vi "OCU_Lyras.vi"(9 "Overview Image Ref In":T7, 10 "at":T6="LPB Pool", 11 "Location of THINK":T11="127.0.0.1") -> ()   [LabVIEW 2013]
doc: "This is the current implementation of the operator control unit (OCU) for sailbot interfacing with this OCU over a network connection. The following features are currently implemented:\n- override control of the rudden angle and sail value by control interface or using keys\n- ability to add missions before and during a run, by clicking and by using GPS location of the boat or an auxiliary GPS attached to the OCU computer\n- modification of tuning values used on the boat\n- indicators for all relevant system status information\n\nAuthors: Jared Kirschner, Jason Curtis"
uses:
  trunk/Software/2-Think/2 Typedefs/sail setpt.ctl
  trunk/Software/2-Think/2 Typedefs/rudder angle.ctl
  trunk/Software/2-Think/2 Typedefs/setpoints to boat.ctl
  trunk/Software/0x2-OCU-Think Comm/0x2 Typedefs/manual override.ctl
  trunk/Software/2-Think/2 Typedefs/eStopCommand.ctl
  trunk/Software/0x2-OCU-Think Comm/0x2 Typedefs/Current Waypoint.ctl
  cRIO_Code/Data/TypeDefs/UTM Location.ctl
  RIO-OCU_Comm/NetworkStreams/Reader/NetworkStreamReader.lvclass
  RIO-OCU_Comm/NetworkStreams/Reader/readType.ctl
  trunk/Software/0x2-OCU-Think Comm/0x2 Typedefs/ocuMessage.ctl
  trunk/Software/0x2-OCU-Think Comm/0x2 Typedefs/ocuCommands.ctl
  RIO-OCU_Comm/NetworkStreams/Writer/NetworkStreamWriter.lvclass
  trunk/Software/2-Think/2 Typedefs/indicator LED.ctl
  trunk/Software/2-Think/2 Typedefs/generalized sensor status.ctl
  trunk/Software/2-Think/2 Typedefs/generalized actuator status.ctl
  trunk/Software/2-Think/2 Typedefs/Which Boat.ctl
  trunk/Software/2-Think/2 Typedefs/robot velocity.ctl
  trunk/Software/2-Think/2 Typedefs/heading.ctl
  trunk/Software/2-Think/2 Typedefs/rate of turn.ctl
  trunk/Software/2-Think/2 Typedefs/pitch and roll.ctl
  trunk/Software/2-Think/2 Typedefs/apparent wind.ctl
  trunk/Software/2-Think/2 Typedefs/apparent wind speed.ctl
  trunk/Software/2-Think/2 Typedefs/apparent wind direction.ctl
  trunk/Software/2-Think/2 Typedefs/Velocity.ctl
  trunk/Software/2-Think/2 Typedefs/absolute wind direction.ctl
  trunk/Software/2-Think/2 Typedefs/absolute wind speed.ctl
  trunk/Software/2-Think/2 Typedefs/absolute water current vector.ctl
  trunk/Software/0x2-OCU-Think Comm/0x2 Typedefs/RIO-OCU update controls.ctl
  trunk/Software/0-OCU/0 Typedefs/Mission Type Radio Buttons.ctl
  trunk/Software/2-Think/2 Typedefs/Goodness Fns Indicator.ctl
  trunk/Software/2-Think/2 Typedefs/UTM Circle.ctl
  trunk/Software/2-Think/2 Globals/2 Global.vi
  trunk/Software/2-Think/2 Typedefs/tacking attempt.ctl
  OCU/Location of Think.ctl
  trunk/Software/0x2-OCU-Think Comm/OCUtoSim.vi
  cRIO_Code/Logic/Classes/Missions/GenericMission/GenericMission.lvclass
  trunk/Software/0-OCU/0 Typedefs/Sail Position.ctl
  trunk/Software/0-OCU/0 Typedefs/Rudder Position.ctl
  trunk/Software/0-OCU/0 Typedefs/Apparent Wind Point of Sail.ctl
  cRIO_Code/Data/TypeDefs/ocuWaypoint.ctl
  cRIO_Code/Logic/Classes/Waypoint/Waypoint.lvclass
  cRIO_Code/Data/TypeDefs/Waypoints List.ctl
  trunk/Software/2-Think/2 Typedefs/PI Constants.ctl
  trunk/Software/2-Think/2 Typedefs/Goodness Weightings.ctl
  trunk/Software/0-OCU/0 Typedefs/Maps.ctl
  <vilib>/vision/Image Controls.llb/IMAQ Image.ctl
  trunk/Software/0x2-OCU-Think Comm/0x2 Typedefs/Sail Setting Tuning.ctl
  trunk/Software/0x2-OCU-Think Comm/0x2 Typedefs/Control values.ctl
panel:
  in  "Tab Control":T1(tab)
  out "Sail Position 2":T2 scale=1.0..-1.0
  out "Rudder Position":T3 scale=50.0..-50.0 scale format="%#_2f"
  in  "Mission Entry Type":T4
  in  "Tolerance":dbl=3.0
  in  "Time(s)":dbl=300.0
  out "You are sailing":T5
  out "Battery Voltage":dbl
  out "Connected?":bool caption="Connection Status"
  out "Mission Map":T7(plugin-control)
  out "# of Waypts":i32
  in  "Overlay Font Size":i16=40
  in  "Stop":bool
  in  "Map Mode":enum32{"M[i]ssion Edit", "M[o]nitoring"}(tab)
  in  "Load MDF":bool
  in  "Mission Def Filepath":path caption="MDF (Mission Definition File) path"
  in  "Reset Missions/Waypts":bool
  in  "Save Waypoints\nand PoI":bool
  out "Absolute\nWind\nDirection":dbl
  out "Heading":T8 format="%05.1f"
  in  "Plot Colors":T9={"Target"=3381759, "No Sail"=16711680, "Change"=16756736, "Pure Waypt"=35080, "Pure Wind"=16860, "Combined"=16777228}
  out "Goodness Functions":picture
  out "Apparent Wind Direction\nPoint of Sail":T10 scale=0.0..360.0 scale format="%4d"
  out "Mission Status":string caption="Current Mission\nStatus"
  in  "GPS COM port":refnum<visa-resource-name>="COM1"
  out "Sensor Status":T12
  in  "Enable \nLocal GPS":bool
  out "Local Wind":dbl
  in  "Log message":string caption="Log message (type and press enter)"
  out "Mission Map 2":T7(plugin-control)
  out "# of Waypts 2":i32
  in  "Overlay Font Size 2":i16=40
  in  "Save Image":bool
  in  "OVERRIDE SAIL?":bool
  in  "OVERRIDE RUDDER?":bool
  in  "Globals":T14(tab)
  out "Don't Tip?":bool
  out "Wind Sensor Status":T12
  out "Estimated Error":dbl
  out "Robot Heading":T8 format="%05.1f"
  out "Robot UTM Location":T15 {"North" format="%#_10f"; "East" format="%#_8f"}
  out "Robot Velocity":T16
  out "Robot\nRate of Turn":T17 format="%05.1f"
  out "Robot Pitch/Roll":T18 {"Roll" format="%05.1f"; "Pitch" format="%05.1f"}
  out "Robot Speed (m/s)":dbl
  out "Absolute Wind":T19 {"East" format="%#_5g"}
  out "Apparent Wind Direction":T20
  out "Apparent Wind Speed":T21
  out "Apparent Wind":T22
  out "Crossing Wind":bool
  out "Setpoints to boat":T23
  out "Sail Position":T24
  out "Rudder Angle":T25
  out "Current Waypoint":T26
  in  "Reset to start":bool
  out "Manual Override":T27
  out "Waypoints Array":T28[](array[typedef]) {"UTM Location"."North" format="%#_10f"; "UTM Location"."East" format="%#_8f"}
  out "Waypoints Object Array":T29
  out "Mission Object Array":refnum<class "GenericMission.lvclass">[](array[class])
  out "Global No Sail Circles":T30[](array[typedef])
  in  "Additional inputs":T31(tab)
  in  "To UTM":bool
  in  "Manual Mission Input":enum32{"Drive", "Round", "Pass", "Station"}(tab)
  in  "Waypoint Location":enum32{"0", "1", "2", "3", "4"}(radio)
  in  "Buoy Side":enum32{"Starboard", "Port"}(radio)
  in  "Buoy to Round":enum32{"0", "1", "2", "3", "4"}(radio)
  in  "Starboard Buoy":enum32{"0", "1", "2", "3", "4"}(radio)=enum."1"
  in  "Port Buoy":enum32{"0", "1", "2", "3", "4"}(radio)
  in  "Buoy B":enum32{"0", "1", "2", "3", "4"}(radio)=enum."1"
  in  "Buoy A":enum32{"0", "1", "2", "3", "4"}(radio)
  in  "Add Mission":bool
  in  "Stored Locations Array":T15[](array[typedef])=[{"UTM Zone"=0.0, "Hemisphere"=enum."North", "East"=0.0, "North"=0.0}, {"UTM Zone"=0.0, "Hemisphere"=enum."North", "East"=0.0, "North"=0.0}, {"UTM Zone"=0.0, "Hemisphere"=enum."North", "East"=0.0, "North"=0.0}, {"UTM Zone"=0.0, "Hemisphere"=enum."North", "East"=0.0, "North"=0.0}, {"UTM Zone"=0.0, "Hemisphere"=enum."North", "East"=0.0, "North"=0.0}] {"North" format="%#_10f"; "East" format="%#_8f"}
  in  "Boat to Point 0":bool
  in  "Boat to Point 1":bool
  in  "Boat to Point 2":bool
  in  "Boat to Point 3":bool
  in  "Boat to Point 4":bool
  in  "Local to Point 4":bool
  in  "Local to Point 3":bool
  in  "Local to Point 2":bool
  in  "Local to Point 1":bool
  in  "Local to Point 0":bool
  in  "Which to UTM?":bool[](array[boolean])
  in  "Update Constants":bool
  in  "Tuning Values":T32={"Goodness Weightings"={"Target Importance"=0.8, "No Sail Importance"=1.0, "Change Importance"=0.5, "Pure Waypoint \nImportance"=0.0, "Pure Wind \nImportance"=0.0}, "PI Constants"={"Proportional Gain"=0.5, "Integral Time"=0.0, "Derivative Time"=0.0}, "No Sail Zone\nTuning Quotient"=0.05, "Heading Change Wind Adjustment"=0.2, "Waypoint Tuning Quotient"=1.0, "Let Sail Out on Windcross"=FALSE, "Shift Goal for currents"=TRUE, "Round Buoy Safety"=5.0, "Sail Setting Options"={"Linear\nMode"=FALSE, "Sails Full In Point"=85.0, "Sails Full Out Point"=180.0}, "Defilter Wind Data"=TRUE, "Irons Range"=50.0, "Aggressiveness"=50.0, "Downwind\nRange"=0.5, "Runprotect?"=FALSE, "Run Range"=0.0, "Convincing range"=0.0} {"Aggressiveness" min=0.0 max=1.0; "Sail Setting Options"."Sails Full Out Point" step=0.1; "Sail Setting Options"."Sails Full In Point" step=0.1; "Goodness Weightings"."Pure Wind \nImportance" min=0.0 step=0.2; "Goodness Weightings"."Pure Waypoint \nImportance" min=0.0 step=0.2; "Goodness Weightings"."Change Importance" min=0.0 step=0.2; "Goodness Weightings"."No Sail Importance" min=0.0 step=0.2; "Goodness Weightings"."Target Importance" min=0.0 step=0.2}
  in  "Simulator controls":enum32{"Running", "Paused"}(tab)
  in  "Set Water Current Speed":dbl
  in  "Set Water Current Direction":dbl(knob) scale=0.0..360.0
  in  "Set Wind Speed":dbl=20.0
  in  "Pause Simulator?":bool
  in  "Set Wind Direction":dbl(knob) scale=0.0..360.0
  in  "Move boat?":bool
  in  "Set Boat Heading":dbl(knob) scale=0.0..360.0
  # "PORT"
  # "STARB"
  # "Local GPS"
  # "Note: if THINK\nis on this computer,\nturning on local GPS will do strange things."
  # "inputting missions:\nGo To Waypoint: set tolerance, and click on map.\nRound Buoy Port/Starboard: set tolerance, click.\nPass Between Buoys: Click one buoy location\nand drag to the other.\nStation Keeping: click southwest corner, drag to \nsoutheast corner. A square will be generated.\nTime(s) currently unimplemented.\nGlobal No-Sail Zone: click center of zone, drag to edge of\nzone. A circle with appropriate radius will be created."
  # "As Measured"
  # "Path Planning"
  # "From Planning Functions"
  # "(this is not a cluster because subitems\nare generated in parallel code)"
  # "HOWTO:\n1. save one or more points by moving GPS sensor to point, and pressing buttons below\n2. choose type of mission from tab control\n3. choose saved point(s) to load into mission. other params come from mission map input above\n4. click \"Add Mission\""
  # "Latlong in\nxx.xxxx format"
  # "We assume\nnorth and west"
  # "Latitude is north\nLongitude is east"
  # "Make sure that\nyour cursor\nis not in the\nbox when you\nclick To UTM"
  # "P"
  # "S"
  # "O"
  # "O"
  # "A"
  # "B"
  # "HOWTO:\nchange values here, \nthen hit:"
  # "Note: the direction the current is coming from is opposite\n the dial. This is the direction the current is going to."
  # "When set,\nclick on map\nto move boat"
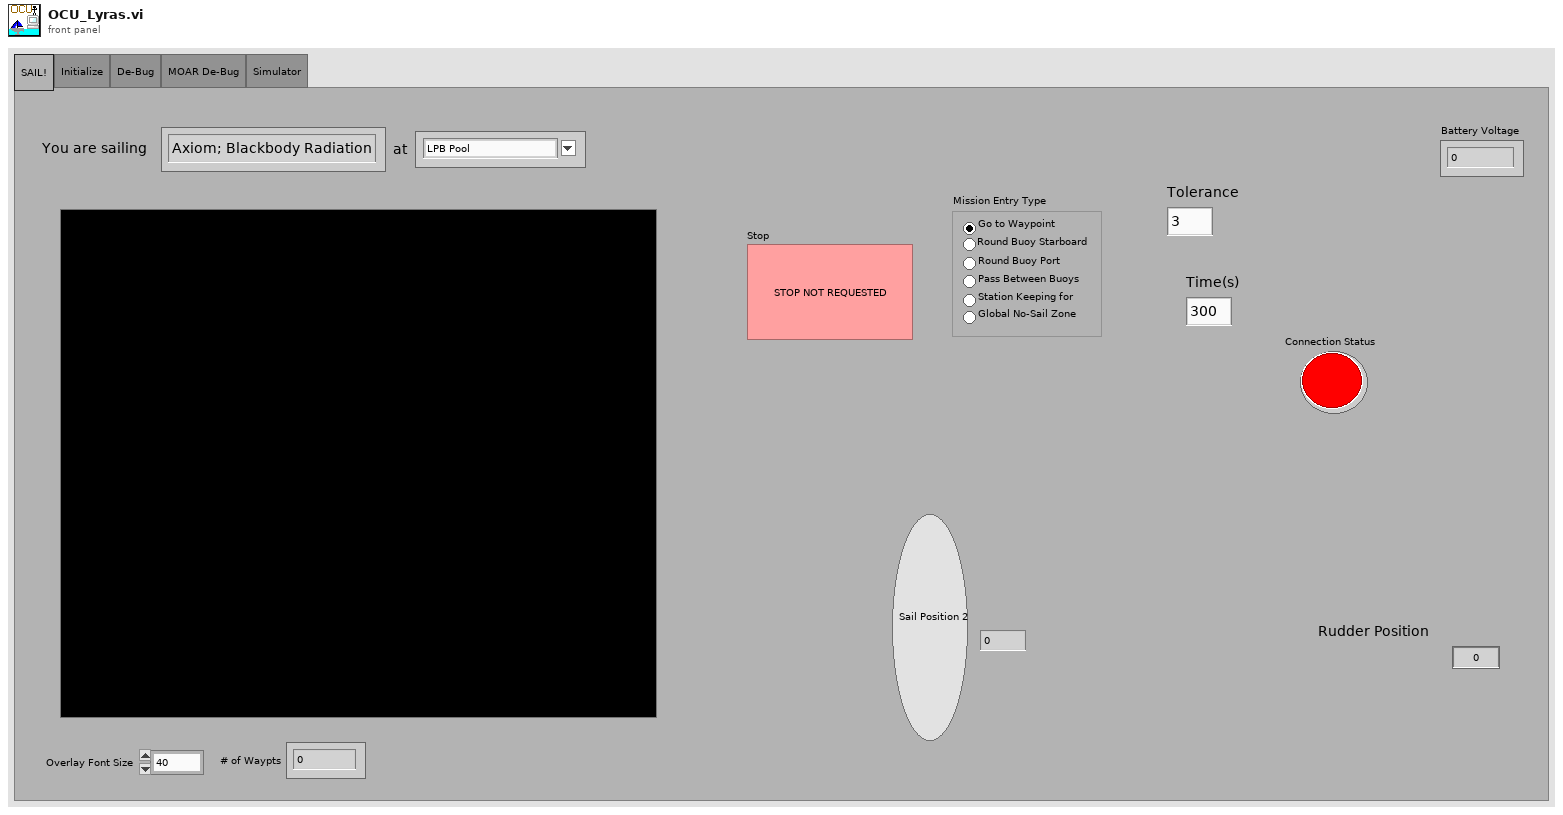
[diagram p1: front panel]
types:
  T1 = enum32{"SAIL!", "Initialize", "De-Bug", "MOAR De-Bug", "Simulator"}
  T2 = typedef "Sail Position.ctl" = dbl
  T3 = typedef "Rudder Position.ctl" = dbl
  T4 = typedef "Mission Type Radio Buttons.ctl" = enum32{"Go to Waypoint", "Round Buoy Starboard", "Round Buoy Port", "Pass Between Buoys", "Station Keeping for", "Global No-Sail Zone"}
  T5 = typedef "Which Boat.ctl" = enum16{"Axiom; Blackbody Radiation", "Simulation"}
  T6 = typedef "Maps.ctl" = string
  T7 = typedef "IMAQ Image.ctl" = refnum<image>
  T8 = typedef "heading.ctl" = dbl
  T9 = cluster{"Target":u32, "No Sail":u32, "Change":u32, "Pure Waypt":u32, "Pure Wind":u32, "Combined":u32}
  T10 = typedef "Apparent Wind Point of Sail.ctl" = dbl
  T11 = typedef "Location of Think.ctl" = string
  T12 = typedef "generalized sensor status.ctl" = cluster{"Sensor Connected":T13, "Sensor Initialized":T13, "Sensor OK":T13, "Latest Error String":string, "GPS Lock":T13}
  T13 = typedef "indicator LED.ctl" = bool
  T14 = enum32{"How Am I", "Where Am I", "What's Around Me", "Path Planning"}
  T15 = typedef "UTM Location.ctl" = cluster{"UTM Zone":dbl, "Hemisphere":enum16{"North", "South"}, "East":dbl, "North":dbl}
  T16 = typedef "robot velocity.ctl" = cluster{"East":dbl, "North":dbl}
  T17 = typedef "rate of turn.ctl" = dbl
  T18 = typedef "pitch and roll.ctl" = cluster{"Pitch":dbl, "Roll":dbl}
  T19 = typedef "Velocity.ctl" = cluster{"East":dbl, "North":dbl}
  T20 = typedef "apparent wind direction.ctl" = dbl
  T21 = typedef "apparent wind speed.ctl" = dbl
  T22 = typedef "apparent wind.ctl" = cluster{"Toward Fore":dbl, "Toward Starboard":dbl}
  T23 = typedef "setpoints to boat.ctl" = cluster{"Sail Position":T24, "Rudder Angle":T25}
  T24 = typedef "sail setpt.ctl" = dbl
  T25 = typedef "rudder angle.ctl" = dbl
  T26 = typedef "Current Waypoint.ctl" = i32
  T27 = typedef "manual override.ctl" = cluster{"Override Active Rudder":bool, "Setpoints":T23, "Override Active Sail":bool}
  T28 = typedef "ocuWaypoint.ctl" = cluster{"Tolerance (m)":dbl, "UTM Location":T15}
  T29 = typedef "Waypoints List.ctl" = refnum<class "Waypoint.lvclass">[]
  T30 = typedef "UTM Circle.ctl" = cluster{"UTM Zone":dbl, "Hemisphere":enum16{"North", "South"}, "East":dbl, "North":dbl, "Radius":dbl}
  T31 = enum32{"Manual Mission Input", "Tuning Constants"}
  T32 = typedef "Control values.ctl" = cluster{"Goodness Weightings":T33, "PI Constants":T34, "No Sail Zone\nTuning Quotient":dbl, "Heading Change Wind Adjustment":dbl, "Waypoint Tuning Quotient":dbl, "Let Sail Out on Windcross":bool, "Shift Goal for currents":bool, "Round Buoy Safety":dbl, "Sail Setting Options":T35, "Defilter Wind Data":bool, "Irons Range":dbl, "Aggressiveness":dbl, "Downwind\nRange":dbl, "Runprotect?":bool, "Run Range":dbl, "Convincing range":dbl}
  T33 = typedef "Goodness Weightings.ctl" = cluster{"Target Importance":dbl, "No Sail Importance":dbl, "Change Importance":dbl, "Pure Waypoint \nImportance":dbl, "Pure Wind \nImportance":dbl}
  T34 = typedef "PI Constants.ctl" = cluster{"Proportional Gain":dbl, "Integral Time":dbl, "Derivative Time":dbl}
  T35 = typedef "Sail Setting Tuning.ctl" = cluster{"Linear\nMode":bool, "Sails Full In Point":dbl, "Sails Full Out Point":dbl}
  T36 = typedef "RIO-OCU update controls.ctl" = cluster{"Sensor Status":T12, "Battery Voltage":dbl, "Rudder Actuator Status":T37, "Sail Actuator Status":T37, "Which Boat Am I?":T5, "Robot Velocity":T16, "Robot UTM Location":T15, "Robot\nHeading ":T8, "Robot\nRate of Turn":T17, "Robot Pitch/Roll":T18, "Apparent Wind":T22, "Apparent Wind\nSpeed":T21, "Apparent Wind\nDirection (º)":T20, "Absolute Wind":T19, "Absolute Wind\nDirection (º)":T38, "Absolute Wind\nSpeed":T39, "Absolute Water Current Vector":T40, "Rudder Angle":T25, "Sail Position":T24, "Manual Override Cluster":T27, "Setpoints to boat":T23, "Current Waypoint":T26, "Think freq.":dbl, "Sense freq.":dbl, "Act freq.":dbl, "E-stop freq.":dbl, "Network \nfreq.":dbl, "Network \nLoop Iterations":i64, "E-Stop":bool, "Serialized Waypoint Array":string, "Serialized Mission Queue Elements":string, "Goodness Functions":T41, "Global No Sail Circles":T30[], "Optimal Heading":dbl, "Crossing Wind":bool, "Estimated Error":dbl, "Don't Tip?":bool, "Tacking Attempt":T42}
  T37 = typedef "generalized actuator status.ctl" = cluster{"Actuator Connected":T13}
  T38 = typedef "absolute wind direction.ctl" = dbl
  T39 = typedef "absolute wind speed.ctl" = dbl
  T40 = typedef "absolute water current vector.ctl" = cluster{"Direction":T20, "Magnitude":T20}
  T41 = typedef "Goodness Fns Indicator.ctl" = cluster{dbl, dbl, dbl[][]}
  T42 = typedef "tacking attempt.ctl" = cluster{"attempting tack":bool, "tacking attempt\ntime remaining":dbl}
  T43 = typedef "0-Image Descriptor.ctl" = cluster{"Upper-Left Corner Coordinates":T15, "Meters/Pixel":dbl}
  T44 = typedef "eStopCommand.ctl" = enum16{"Reset E-Stop", "Get E-Stop", "Set E-Stop"}
  T45 = typedef "ocuMessage.ctl" = cluster{"OCU Command":T46, "Data":variant}
  T46 = typedef "ocuCommands.ctl" = enum16{"Pass", "Send override", "Set waypoint number", "Stop", "Add Mission", "Reset Missions/Waypts", "Edit Control Values", "Add Global No-Sail", "Log Message"}
  T47 = enum8{"Enabled", "Disabled", "Disabled and Grayed Out"}
  T48 = typedef "eventvkey.ctl" = enum16{"ASCII", "Enter", "Return", "Shift", "Ctrl", "Alt", "Cmd", "Opt", "Caps", "NumLock", "Clear", "Break", "Up", "Down", "Left", "Right", "Insert", "Delete", "Home", "End", "PageUp", "PageDown", "Escape", "Help", "Pause", "ScrollLock", "F1", "F2", "F3", "F4", "F5", "F6", "F7", "F8", "F9", "F10", "F11", "F12", "F13", "F14", "F15", "F16", "F17", "F18", "F19", "F20", "F21", "F22", "F23", "F24", "Play", "VolumeUp", "VolumeDown", "Mute", "Two Byte Char"}
  T49 = typedef "NetworkStreamReader.lvclass/readType.ctl" = enum16{"Next in buffer", "Most current"}
  T50 = cluster{"Image Ref Out":T7, "Image Descriptor":T43}
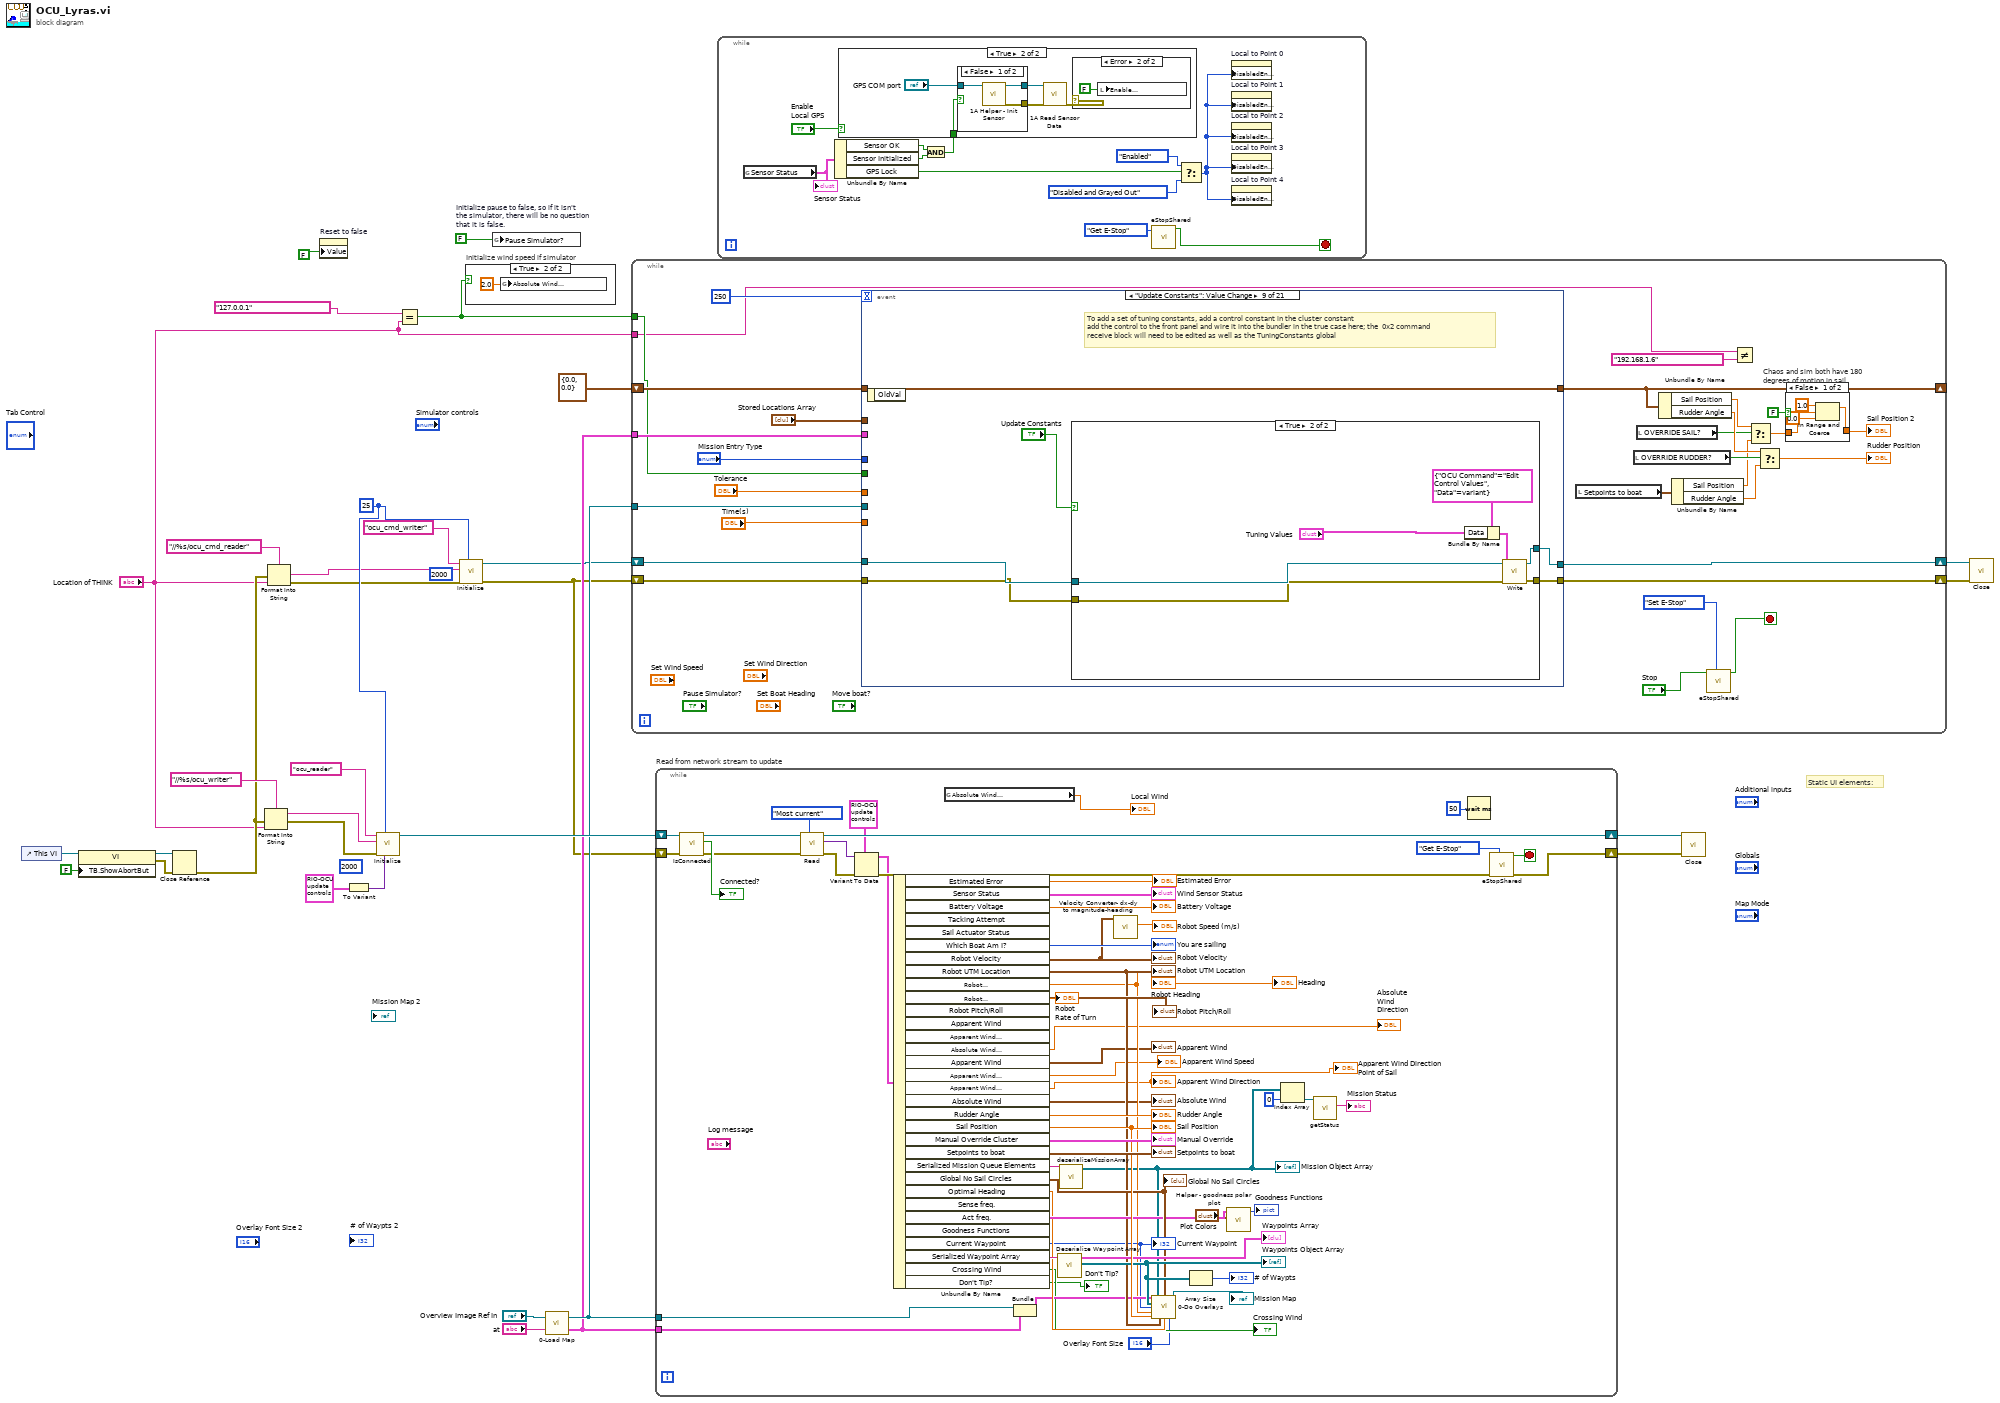
[diagram p0: block diagram]
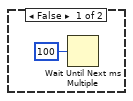
[diagram p3: hidden frame]
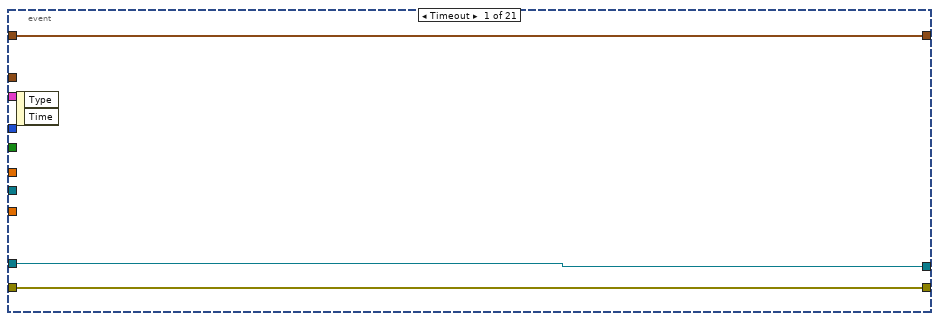
[diagram p7: hidden frame]
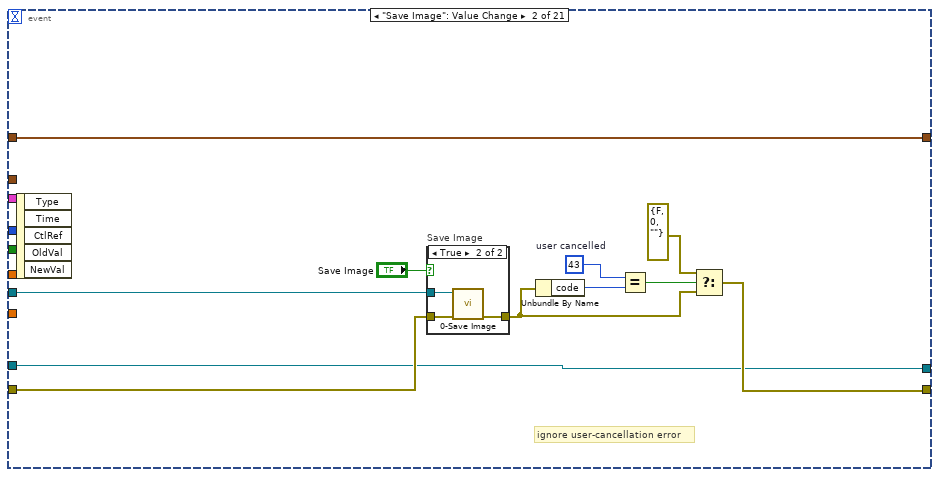
[diagram p8: hidden frame]
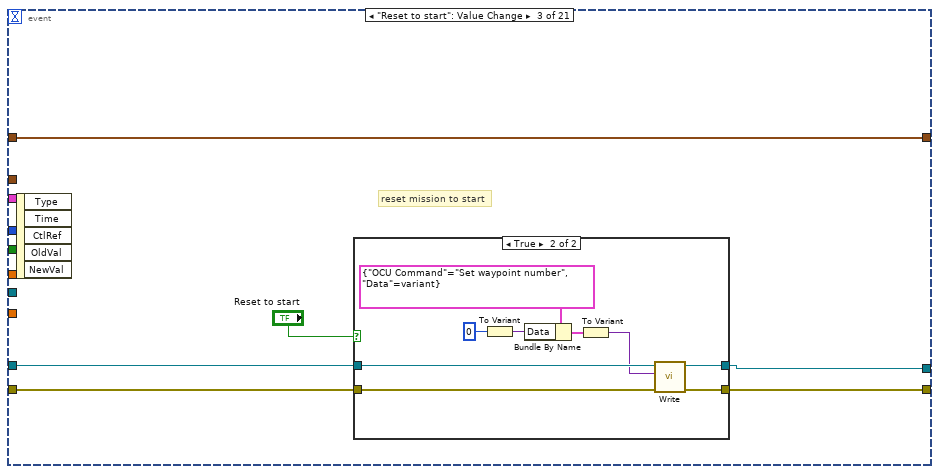
[diagram p10: hidden frame]
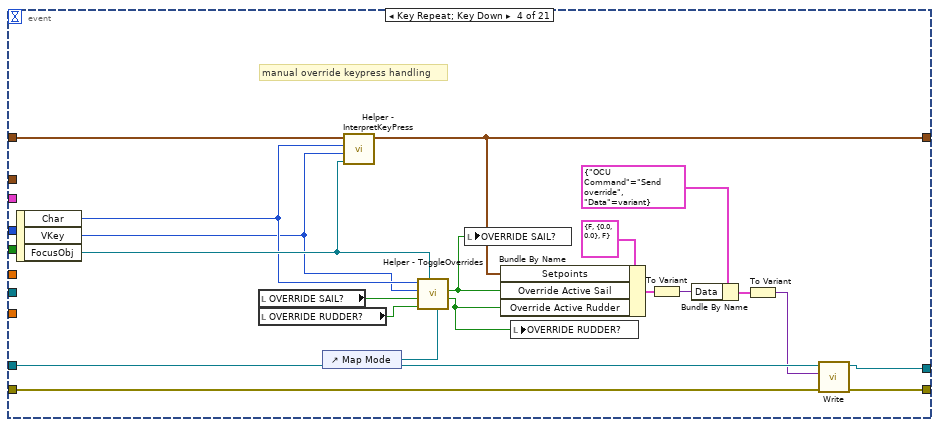
[diagram p12: hidden frame]
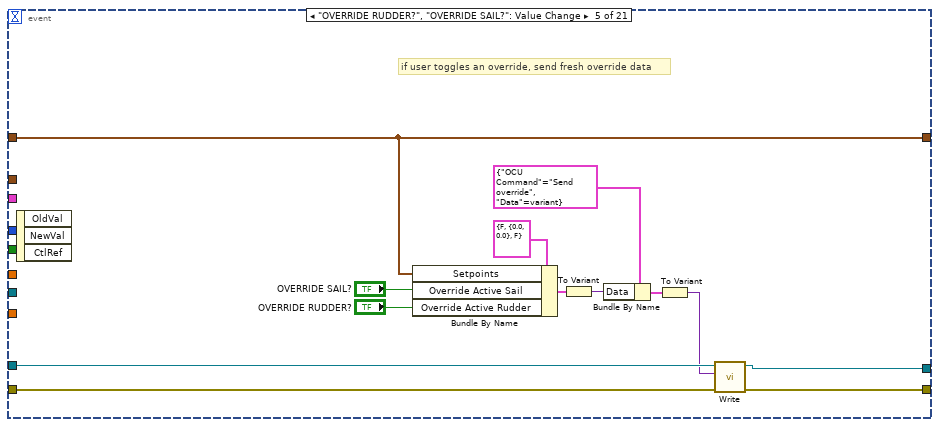
[diagram p13: hidden frame]
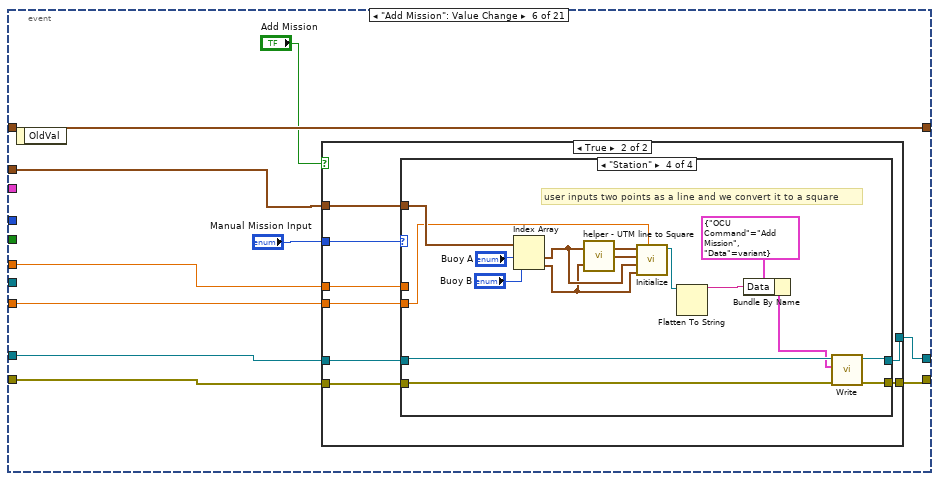
[diagram p14: hidden frame]
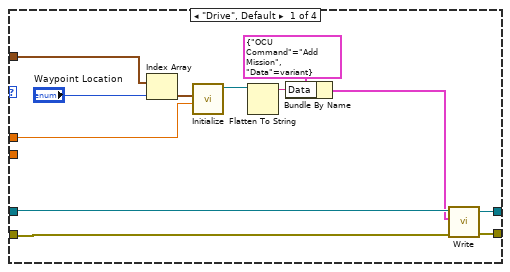
[diagram p16: hidden frame]
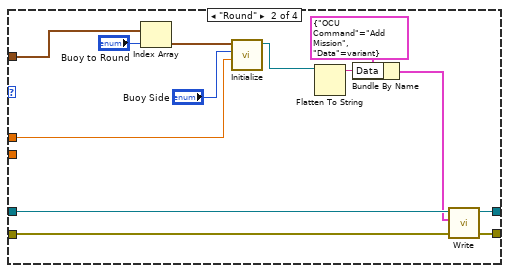
[diagram p17: hidden frame]
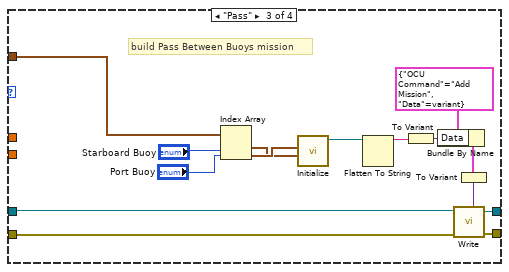
[diagram p18: hidden frame]
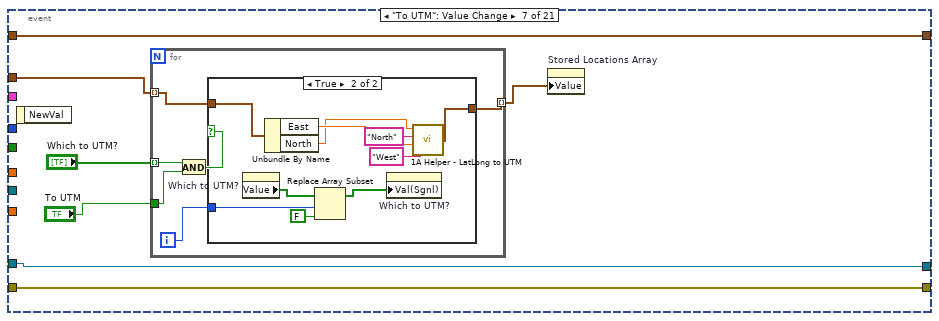
[diagram p19: hidden frame]
diagram:
  w4 = FALSE  # Initialize pause to false, so if it isn't the simulator, there will be no question that it is false.
  (unwired) 2000 ("connection timeout")
  (unwired) 2000 ("connection timeout")
  w31 = 25 ("writer buffer size")
  # "Static UI elements:"
  n1 = control-ref of="This VI"() -> (w22:refnum<vi>)
  n2 = property class="VI"(reference=w22, "TB.ShowAbortBut"=FALSE ("Tool Bar:Show Abort Button")) -> (reference out=w20:refnum<vi>, error out=w19:errorcluster)  [unwired: 1 in]
  n3 = Close Reference(reference=w20, error in (no error)=w19) -> (error out=w18:errorcluster)
  n4 = Format Into String(format string="//%s/ocu_writer", error in=w18, "Location of THINK") -> (resulting string=w12:string, error out=w16:errorcluster)  [unwired: 1 in]
  n5 = Format Into String(format string="//%s/ocu_cmd_reader", error in=w18, "Location of THINK") -> (resulting string=w10:string, error out=w17:errorcluster)  [unwired: 1 in]
  n6 = property on="Reset to false" class="Bool (strict)"("Value"=FALSE ("Pause Simulator?")) -> ()  [unwired: 2 in, 2 out]
  n7 = To Variant(anything=T36 {"Sensor Status"={"Sensor Connected"=FALSE, "Sensor Initialized"=FALSE, "Sensor OK"=FALSE, "Latest Error String"="", "GPS Lock"=FALSE}, "Battery Voltage"=0.0, "Rudder Actuator Status"={"Actuator Connected"=FALSE}, "Sail Actuator Status"={"Actuator Connected"=FALSE}, "Which Boat Am I?"=enum."Axiom; Blackbody Radiation", "Robot Velocity"={"East"=0.0, "North"=0.0}, "Robot UTM Location"={"UTM Zone"=0.0, "Hemisphere"=enum."North", "East"=0.0, "North"=0.0}, "Robot\nHeading "=0.0, "Robot\nRate of Turn"=0.0, "Robot Pitch/Roll"={"Pitch"=0.0, "Roll"=0.0}, "Apparent Wind"={"Toward Fore"=0.0, "Toward Starboard"=0.0}, "Apparent Wind\nSpeed"=0.0, "Apparent Wind\nDirection (º)"=0.0, "Absolute Wind"={"East"=0.0, "North"=0.0}, "Absolute Wind\nDirection (º)"=0.0, "Absolute Wind\nSpeed"=0.0, "Absolute Water Current Vector"={"Direction"=0.0, "Magnitude"=0.0}, "Rudder Angle"=0.0, "Sail Position"=0.0, "Manual Override Cluster"={"Override Active Rudder"=FALSE, "Setpoints"={"Sail Position"=0.0, "Rudder Angle"=0.0}, "Override Active Sail"=FALSE}, "Setpoints to boat"={"Sail Position"=0.0, "Rudder Angle"=0.0}, "Current Waypoint"=0, "Think freq."=0.0, "Sense freq."=0.0, "Act freq."=0.0, "E-stop freq."=0.0, "Network \nfreq."=0.0, "Network \nLoop Iterations"=0, "E-Stop"=FALSE, "Serialized Waypoint Array"="", "Serialized Mission Queue Elements"="", "Goodness Functions"={0.0, 0.0, []}, "Global No Sail Circles"=[], "Optimal Heading"=0.0, "Crossing Wind"=FALSE, "Estimated Error"=0.0, "Don't Tip?"=FALSE, "Tacking Attempt"={"attempting tack"=FALSE, "tacking attempt\ntime remaining"=0.0}} ("RIO->OCU update data")) -> (Variant=w30:variant)
  n8 = call "Initialize.vi"("Default return"=w30, "reader buffer size"=w31, "error in (no error)"=w16, "writer url"=w12, "reader name"="ocu_reader" ("writer name")) -> ("NetworkStreamWriter out"=w32:refnum<class "NetworkStreamReader.lvclass">)  [unwired: 5 in, 1 out]
  n9 = Equal?(x=T11 "127.0.0.1" ("y"), y="Location of THINK") -> (x = y?=w3:bool)
  n10 = call "Initialize.vi"("writer buffer size"=w31, "error in (no error)"=w17, "reader url"=w10, "writer name"="ocu_cmd_writer") -> ("error out"=w6:errorcluster, "NetworkStreamWriter out"=w7:refnum<class "NetworkStreamWriter.lvclass">)  [unwired: 6 in]
  n11 = case "Initialize wind speed if simulator" shown="True" w3 {
    frame False {
    }
    frame True {
      n12 = global write "2 Global.vi" "Absolute Wind\nSpeed"(T39 2.0 ("Absolute Wind\nSpeed")) -> ()
    }
  }
  n13 = global write "OCUtoSim.vi" "Pause Simulator?"(w4) -> ()
  n14 = call "0-Load Map.vi"("Map Name"="at", "Image Ref In"="Overview Image Ref In") -> ("Image Descriptor"=w14:T43, "Image Ref Out"=w27:T7)
  n15 = while {
    shift-right: [w63] -> w23
    shift-left: w6 -> [w46]
    shift-right: [w57] -> _
    shift-left: T23 {"Sail Position"=0.0, "Rudder Angle"=0.0} ("Setpoints") -> [w64]
    shift-right: [w59] -> w24
    shift-left: w7 -> [w47]
    tunnel: w27 -> [w58]
    tunnel: w14 -> [w56]
    tunnel: w3 -> [w41]
    tunnel: "Location of THINK" -> [w38]
    stop <- w62 stop-if-true
    n16 = event shown="[8] \"Update Constants\": Value Change" {
      selector: _ -> [_ _ _ _ _ _ _ _ _ _ _ _ _ _ _ _ _ _ _ _ _]
      dyn-events: _ -> [_ _ _ _ _ _ _ _ _ _ _ _ _ _ _ _ _ _ _ _ _]
      timeout: 250 -> [_ _ _ _ _ _ _ _ _ _ _ _ _ _ _ _ _ _ _ _ _]
      tunnel: w64 -> [w72 w79 w93 w125 w128 w146 w218 w246 w270 w292 w308 w317 w358 w368 w392 w538 w545 w554 w564 w576 w581]
      tunnel: [w72 w79 w93 w123 w128 w146 w218 w246 w270 w292 w308 w317 w358 w368 w392 w538 w545 w554 w564 w576 w581] -> w57
      tunnel: w46 -> [w70 w77 w90 w120 w135 w147 w219 w244 w267 w284 w307 w315 w356 w369 w391 w536 w543 w552 w562 w574 w583]
      tunnel: [w70 w74 w88 w119 w134 w144 w219 w244 w265 w282 w307 w314 w354 w369 w389 w536 w543 w552 w562 w574 w583] -> w63
      tunnel: w47 -> [w71 w73 w91 w122 w137 w148 w220 w245 w268 w283 w306 w313 w357 w370 w387 w537 w544 w553 w563 w575 w582]
      tunnel: [w71 w73 w89 w121 w136 w143 w220 w245 w266 w285 w306 w312 w355 w370 w388 w537 w544 w553 w563 w575 w582] -> w59
      tunnel: w58 -> [_ w78 _ _ _ _ _ _ _ _ _ _ _ _ _ _ _ _ _ _ _]
      tunnel: w56 -> [_ _ _ _ _ _ _ _ _ _ _ _ _ _ w390 _ _ _ _ _ _]
      tunnel: "Mission Entry Type" -> [_ _ _ _ _ _ _ _ _ _ _ _ _ _ w386 _ _ _ _ _ _]
      tunnel: "Tolerance" -> [_ _ _ _ _ w145 _ _ _ _ _ _ _ _ w385 _ _ _ _ _ _]
      tunnel: "Time(s)" -> [_ _ _ _ _ w140 _ _ _ _ _ _ _ _ w384 _ _ _ _ _ _]
      tunnel: w41 -> [_ _ _ _ _ _ _ _ _ _ _ _ _ _ _ w534 w548 w558 w561 w578 w588]
      tunnel: "Stored Locations Array" -> [_ _ _ _ _ w139 w217 _ _ _ _ _ _ _ _ _ _ _ _ _ _]
      event Timeout {
        n17 = event-data() -> ()  [unwired: 1 in, 2 out]
      }
      event "Save Image": Value Change {
        w82 = 43  # user cancelled
        # "ignore user-cancellation error"
        n18 = event-data() -> ()  [unwired: 1 in, 5 out]
        n19 = case "Save Image" shown="True" "Save Image" {
          tunnel: w77 -> [w84 w87]
          tunnel: [w84 w86] -> w76
          tunnel: w78 -> [_ w85]
          frame False {
          }
          frame True {
            n20 = call "0-Save Image.vi"("Error In"=w87, "Image in"=w85) -> ("Error Out"=w86:errorcluster)  [unwired: 9 in]
          }
        }
        n21 = Unbundle By Name(w76) -> ("code"=w83:i32)
        n22 = Equal?(x=w82, y=w83) -> (x = y?=w81:bool)
        n23 = Select(t=errorcluster {"status"=FALSE, "code"=0, "source"=""}, s=w81, f=w76) -> (s? t:f=w74:errorcluster)
      }
      event "Reset to start": Value Change {
        # "reset mission to start"
        n24 = event-data() -> ()  [unwired: 1 in, 5 out]
        n25 = case shown="True" "Reset to start" {
          tunnel: w91 -> [w95 w101]
          tunnel: w90 -> [w94 w102]
          tunnel: [w95 w104] -> w89
          tunnel: [w94 w103] -> w88
          frame False {
          }
          frame True {
            n26 = To Variant(anything=T26 0 ("Current Waypoint")) -> (Variant=w99:variant)
            n27 = Bundle By Name(cluster=T45 {"OCU Command"=enum."Set waypoint number", "Data"=variant}, "Data"=w99) -> (w97:T45)
            n28 = To Variant(anything=w97) -> (Variant=w96:variant)
            n29 = call "Write.vi"("error in (no error)"=w102, "element"=w96, "NetworkStreamWriter in"=w101) -> ("error out"=w103:errorcluster, "NetworkStreamWriter out"=w104:refnum<class "NetworkStreamWriter.lvclass">)  [unwired: 7 in]
          }
        }
      }
      event Key Repeat; Key Down {
        # "manual override keypress handling"
        n30 = event-data() -> ("Char"=w112:i16, "VKey"=w111:T48, "FocusObj"=w113:refnum<vi>)  [unwired: 1 in]
        n31 = local read "OVERRIDE SAIL?"() -> (w110:bool)
        n32 = local read "OVERRIDE RUDDER?"() -> (w109:bool)
        n33 = control-ref of="Map Mode"() -> (w105:refnum<vi>)
        n34 = call "Helper - InterpretKeyPress.vi"("FocusObj"=w113, "VKey"=w111, "Char"=w112, "Command In"=w125) -> ("Command Out"=w123:T23)  [unwired: 7 in]
        n35 = call "Helper - ToggleOverrides.vi"("Map Mode Tab Control Ref"=w105, "FocusObj"=w113, "Rudder Override?"=w109, "Sail Override?"=w110, "VKey"=w111, "Char"=w112) -> ("Override Rudder"=w108:bool, "Override Sail"=w107:bool, "OCU Tab Control Ref"=w106:refnum<vi>)  [unwired: 3 in]
        n36 = local write "OVERRIDE SAIL?"(w107) -> ()
        n37 = Bundle By Name(cluster=T27 {"Override Active Rudder"=FALSE, "Setpoints"={"Sail Position"=0.0, "Rudder Angle"=0.0}, "Override Active Sail"=FALSE} ("Manual Override Cluster"), "Setpoints"=w123, "Override Active Sail"=w107, "Override Active Rudder"=w108) -> (w115:T27)
        n38 = local write "OVERRIDE RUDDER?"(w108) -> ()
        n39 = To Variant(anything=w115) -> (Variant=w118:variant)
        n40 = Bundle By Name(cluster=T45 {"OCU Command"=enum."Send override", "Data"=variant}, "Data"=w118) -> (w117:T45)
        n41 = To Variant(anything=w117) -> (Variant=w114:variant)
        n42 = call "Write.vi"("error in (no error)"=w120, "element"=w114, "NetworkStreamWriter in"=w122) -> ("error out"=w119:errorcluster, "NetworkStreamWriter out"=w121:refnum<class "NetworkStreamWriter.lvclass">)  [unwired: 7 in]
      }
      event "OVERRIDE RUDDER?", "OVERRIDE SAIL?": Value Change {
        # "if user toggles an override, send fresh override data"
        n43 = event-data() -> ()  [unwired: 1 in, 3 out]
        n44 = Bundle By Name(cluster=T27 {"Override Active Rudder"=FALSE, "Setpoints"={"Sail Position"=0.0, "Rudder Angle"=0.0}, "Override Active Sail"=FALSE} ("Manual Override Cluster"), "Setpoints"=w128, "Override Active Sail"="OVERRIDE SAIL?", "Override Active Rudder"="OVERRIDE RUDDER?") -> (w130:T27)
        n45 = To Variant(anything=w130) -> (Variant=w133:variant)
        n46 = Bundle By Name(cluster=T45 {"OCU Command"=enum."Send override", "Data"=variant}, "Data"=w133) -> (w132:T45)
        n47 = To Variant(anything=w132) -> (Variant=w129:variant)
        n48 = call "Write.vi"("error in (no error)"=w135, "element"=w129, "NetworkStreamWriter in"=w137) -> ("error out"=w134:errorcluster, "NetworkStreamWriter out"=w136:refnum<class "NetworkStreamWriter.lvclass">)  [unwired: 7 in]
      }
      event "Add Mission": Value Change {
        n49 = event-data() -> ()  [unwired: 1 in, 1 out]
        n50 = case shown="True" "Add Mission" {
          tunnel: w148 -> [w150 w158]
          tunnel: w147 -> [w149 w157]
          tunnel: w145 -> [_ w156]
          tunnel: [w149 w155] -> w144
          tunnel: [w150 w154] -> w143
          tunnel: "Manual Mission Input" -> [_ w153]
          tunnel: w139 -> [_ w152]
          tunnel: w140 -> [_ w151]
          frame False {
          }
          frame True {
            n51 = case shown="\"Station\"" w153 {
              tunnel: w157 -> [w166 w179 w188 w206]
              tunnel: [w170 w179 w191 w211] -> w155
              tunnel: w156 -> [w167 w182 _ _]
              tunnel: [w169 w181 w192 w212] -> w154
              tunnel: w158 -> [w168 w180 w193 w210]
              tunnel: w152 -> [w161 w177 w187 w205]
              tunnel: w151 -> [_ _ _ w198]
              frame "Drive", Default {
                n52 = Index Array(array=w161, index="Waypoint Location") -> (element=w164:T15)
                n53 = call "Initialize.vi"("Tolerance (m)"=w167, "Drive Location"=w164) -> ("Drive out"=w162:refnum<class "DriveTo.lvclass">)  [unwired: 8 in, 1 out]
                n54 = Flatten To String(anything=w162) -> (data string=w160:string)  [unwired: 3 in, 2 out]
                n55 = Bundle By Name(cluster=T45 {"OCU Command"=enum."Add Mission", "Data"=variant}, "Data"=w160) -> (w159:T45)
                n56 = call "Write.vi"("error in (no error)"=w166, "element"=w159, "NetworkStreamWriter in"=w168) -> ("error out"=w170:errorcluster, "NetworkStreamWriter out"=w169:refnum<class "NetworkStreamWriter.lvclass">)  [unwired: 7 in]
              }
              frame "Round" {
                n57 = Index Array(array=w177, index="Buoy to Round") -> (element=w176:T15)
                n58 = call "Initialize.vi"("Tolerance (m)"=w182, "Round side?"="Buoy Side", "Buoy to Round"=w176) -> ("RoundBuoys out"=w171:refnum<class "RoundBuoy.lvclass">)  [unwired: 7 in, 1 out]
                n59 = Flatten To String(anything=w171) -> (data string=w173:string)  [unwired: 3 in, 2 out]
                n60 = Bundle By Name(cluster=T45 {"OCU Command"=enum."Add Mission", "Data"=variant}, "Data"=w173) -> (w172:T45)
                n61 = call "Write.vi"("element"=w172, "NetworkStreamWriter in"=w180) -> ("NetworkStreamWriter out"=w181:refnum<class "NetworkStreamWriter.lvclass">)  [unwired: 8 in, 1 out]
              }
              frame "Pass" {
                # "build Pass Between Buoys mission"
                n62 = Index Array(array=w187, index #1="Starboard Buoy", index #2="Port Buoy") -> (element #1=w183:T15, element #2=w184:T15)
                n63 = call "Initialize.vi"("Buoy Pass 2"=w183, "Buoy Pass 1"=w184) -> ("PassBuoys out"=w189:refnum<class "PassBuoys.lvclass">)  [unwired: 8 in, 1 out]
                n64 = Flatten To String(anything=w189) -> (data string=w195:string)  [unwired: 3 in, 2 out]
                n65 = To Variant(anything=w195) -> (Variant=w196:variant)
                n66 = Bundle By Name(cluster=T45 {"OCU Command"=enum."Add Mission", "Data"=variant}, "Data"=w196) -> (w194:T45)
                n67 = To Variant(anything=w194) -> (Variant=w190:variant)
                n68 = call "Write.vi"("error in (no error)"=w188, "element"=w190, "NetworkStreamWriter in"=w193) -> ("error out"=w191:errorcluster, "NetworkStreamWriter out"=w192:refnum<class "NetworkStreamWriter.lvclass">)  [unwired: 7 in]
              }
              frame "Station" {
                # "user inputs two points as a line and we convert it to a square"
                n69 = Index Array(array=w205, index #1="Buoy A", index #2="Buoy B") -> (element #1=w202:T15, element #2=w201:T15)
                n70 = call "helper - UTM line to Square.vi"("Endpoint 2, UTM"=w201, "Endpoint 1, UTM"=w202) -> ("Endpoint 4, UTM"=w208:T15, "Endpoint 3, UTM"=w207:T15)
                n71 = call "Initialize.vi"("Duration (s)"=w198, "Buoy SE"=w201, "Buoy SW"=w202, "Buoy NE"=w208, "Buoy NW"=w207) -> ("StationKeeping out"=w209:refnum<class "StationKeeping.lvclass">)  [unwired: 5 in, 1 out]
                n72 = Flatten To String(anything=w209) -> (data string=w200:string)  [unwired: 3 in, 2 out]
                n73 = Bundle By Name(cluster=T45 {"OCU Command"=enum."Add Mission", "Data"=variant}, "Data"=w200) -> (w199:T45)
                n74 = call "Write.vi"("error in (no error)"=w206, "element"=w199, "NetworkStreamWriter in"=w210) -> ("error out"=w211:errorcluster, "NetworkStreamWriter out"=w212:refnum<class "NetworkStreamWriter.lvclass">)  [unwired: 7 in]
              }
            }
          }
        }
      }
      event "To UTM": Value Change {
        n75 = event-data() -> ()  [unwired: 1 in, 1 out]
        n76 = for {
          tunnel: w217 -> [w226] mode=indexing
          tunnel: "Which to UTM?" -> [w224] mode=indexing
          tunnel: [w225] -> w215 mode=indexing
          tunnel: "To UTM" -> [w222]
          i -> [w221]
          n77 = And(x=w224, y=w222) -> (x .and. y?=w223:bool)
          n78 = case shown="True" w223 {
            tunnel: w226 -> [w227 w235]
            tunnel: [w227 w234] -> w225
            tunnel: w221 -> [_ w231]
            frame False {
            }
            frame True {
              n79 = property on="Which to UTM?" class="Arr (strict)"() -> ("Value"=w230:bool[])  [unwired: 2 in, 2 out]
              n80 = Unbundle By Name(w235) -> ("East"=w233:dbl, "North"=w232:dbl)
              n81 = Replace Array Subset(array=w230, new element=FALSE ("new element/subarray"), index=w231) -> (w228:bool[])
              n82 = property on="Which to UTM?" class="Arr (strict)"("Val(Sgnl)"=w228) -> ()  [unwired: 2 in, 2 out]
              n83 = call "1A Helper - LatLong to UTM.vi"("East/West"="West", "Longitude"=w233, "North/South"="North", "Latitude"=w232) -> ("Robot UTM Location"=w234:T15)
            }
          }
        }
        n84 = property on="Stored Locations Array" class="Arr (strict)"("Value"=w215) -> ()  [unwired: 2 in, 2 out]
      }
      event "Boat to Point 0", "Boat to Point 1", "Boat to Point 2", "Boat to Point 3", "Boat to Point 4", "Local to Point 3", "Local to Point 2", "Local to Point 1", "Local to Point 0", "Local to Point 4": Value Change {
        # "save the current GPS location to one of the saved points."
        n85 = event-data() -> ()  [unwired: 1 in, 1 out]
        n86 = Build Array("Boat to Point 0", "Boat to Point 1", "Boat to Point 2", "Boat to Point 3", "Boat to Point 4") -> (w247:bool[])
        n87 = Build Array("Local to Point 0", "Local to Point 1", "Local to Point 2", "Local to Point 3", "Local to Point 4") -> (w238:bool[])
        n88 = for {
          tunnel: w247 -> [w260] mode=indexing
          i -> [w259]
          n89 = case shown="True" w260 {
            tunnel: w259 -> [_ w262]
            frame False {
            }
            frame True {
              # "load from boat GPS"
              n90 = local read "Stored Locations Array"() -> (w264:T15[])
              n91 = local read "Robot UTM Location"() -> (w261:T15)
              n92 = Replace Array Subset(array=w264, new element=w261, index=w262) -> (w263:T15[])
              n93 = local write "Stored Locations Array"(w263) -> ()
            }
          }
        }
        n94 = for {
          tunnel: w238 -> [w254] mode=indexing
          i -> [w253]
          n95 = case shown="True" w254 {
            tunnel: w253 -> [_ w255]
            frame False {
            }
            frame True {
              # "load from local GPS"
              n96 = local read "Stored Locations Array"() -> (w257:T15[])
              n97 = global read "2 Global.vi" "Robot UTM Location"() -> (w256:T15)
              n98 = Replace Array Subset(array=w257, new element=w256, index=w255) -> (w258:T15[])
              n99 = local write "Stored Locations Array"(w258) -> ()
            }
          }
        }
      }
      event "Update Constants": Value Change {
        # "To add a set of tuning constants, add a control constant in the cluster constant\nadd the control to the front panel and wire it into the bundler in the true case here; the  0x2 command\nreceive block will need to be edited as well as the TuningConstants global"
        n100 = event-data() -> ()  [unwired: 1 in, 1 out]
        n101 = case shown="True" "Update Constants" {
          tunnel: w268 -> [w272 w278]
          tunnel: w267 -> [w271 w277]
          tunnel: [w272 w276] -> w266
          tunnel: [w271 w275] -> w265
          frame False {
          }
          frame True {
            n102 = Bundle By Name(cluster=T45 {"OCU Command"=enum."Edit Control Values", "Data"=variant}, "Data"="Tuning Values") -> (w274:T45)
            n103 = call "Write.vi"("error in (no error)"=w277, "element"=w274, "NetworkStreamWriter in"=w278) -> ("error out"=w275:errorcluster, "NetworkStreamWriter out"=w276:refnum<class "NetworkStreamWriter.lvclass">)  [unwired: 7 in]
          }
        }
      }
      event #9 (no event record) {
        # "Remove carriage\nreturn."
        # "Enter key?"
        n104 = event-data() -> ("ScanCode"=w281)  [unwired: 1 in, 2 out]
        n105 = Equal?(x=w281, y=i16 28) -> (x = y?=w290:bool)
        n106 = Search and Replace String(replace all?=TRUE ("replace all? (F)"), search string="\n" ("string"), replace string="") -> (input string=w280:string, result string=w287:string)  [unwired: 4 in, 3 out]
        n107 = case "Was the log message entered?" shown="True" w290 {
          tunnel: [w294 w303] -> w285
          tunnel: [w293 w302] -> w282
          tunnel: w284 -> [w293 w297]
          tunnel: w283 -> [w294 w301]
          tunnel: w287 -> [_ w298]
          frame False {
          }
          frame True {
            w295 = ""
            n108 = To Variant(anything=w298) -> (Variant=w305:variant)
            n109 = Bundle By Name(cluster=T45 {"OCU Command"=enum."Log Message", "Data"=variant}, "Data"=w305) -> (w304:T45)
            n110 = To Variant(anything=w304) -> (Variant=w299:variant)
            n111 = call "Write.vi"("element"=w299, "NetworkStreamWriter in"=w301) -> ("error out"=w302:errorcluster, "NetworkStreamWriter out"=w303:refnum<class "NetworkStreamWriter.lvclass">, "error in (no error)"=w296:errorcluster)  [unwired: 7 in]
          }
        }
      }
      event "Save Waypoints\nand PoI": Value Change {
        n112 = event-data() -> ()  [unwired: 1 in, 1 out]
        n113 = case "Save MDF" shown="True" "Save Waypoints\nand PoI" {
          frame False {
          }
          frame True {
            n114 = local read "Global No Sail Circles"() -> (w310:T30[])
            n115 = local read "Mission Object Array"() -> (w311:refnum<class "GenericMission.lvclass">[])
            n116 = call "0-Write MDF.vi"("Global No Sail Circles"=w310, "Missions (Object Array)"=w311) -> ()  [unwired: 3 in, 1 out]
          }
        }
      }
      event "Load MDF": Value Change {
        n117 = event-data() -> ()  [unwired: 1 in, 1 out]
        n118 = case "Load MDF" shown="True" "Load MDF" {
          tunnel: w315 -> [w318 w321]
          tunnel: [w318 w328] -> w314
          tunnel: w313 -> [w319 w323]
          tunnel: [w319 w326] -> w312
          frame False {
          }
          frame True {
            w325 = T45 {"OCU Command"=enum."Reset Missions/Waypts", "Data"=variant}  # clear missions
            n119 = To Variant(anything=w325) -> (Variant=w324:variant)
            n120 = call "Write.vi"("error in (no error)"=w321, "element"=w324, "NetworkStreamWriter in"=w323) -> ("error out"=w320:errorcluster, "NetworkStreamWriter out"=w322:refnum<class "NetworkStreamWriter.lvclass">)  [unwired: 7 in]
            n121 = call "0-Read MDF.vi"("Error in"=w320, "MDF file path"="Mission Def Filepath") -> ("Error out"=w330:errorcluster, "Global No Sail Circles"=w332:T30[], "Missions (Object Array)"=w331:refnum<class "GenericMission.lvclass">[])  [unwired: 1 in]
            n122 = for {
              tunnel: w331 -> [w343] mode=indexing
              shift-right: [w349] -> w329
              shift-left: w330 -> [w345]
              shift-right: [w347] -> w327
              shift-left: w322 -> [w348]
              n123 = Flatten To String(anything=w343, error in (no error)=w345) -> (data string=w344:string, error out=w346:errorcluster)  [unwired: 2 in, 1 out]
              n124 = To Variant(anything=w344) -> (Variant=w351:variant)
              n125 = Bundle By Name(cluster=T45 {"OCU Command"=enum."Add Mission", "Data"=variant}, "Data"=w351) -> (w352:T45)
              n126 = To Variant(anything=w352) -> (Variant=w350:variant)
              n127 = call "Write.vi"("error in (no error)"=w346, "element"=w350, "NetworkStreamWriter in"=w348) -> ("error out"=w349:errorcluster, "NetworkStreamWriter out"=w347:refnum<class "NetworkStreamWriter.lvclass">)  [unwired: 7 in]
            }
            n128 = local write "Mission Object Array"(w331) -> ()
            n129 = local write "Global No Sail Circles"(w332) -> ()
            n130 = for {
              tunnel: w332 -> [w335] mode=indexing
              shift-right: [w338] -> w328
              shift-left: w329 -> [w334]
              shift-right: [w336] -> w326
              shift-left: w327 -> [w337]
              n131 = To Variant(anything=w335) -> (Variant=w340:variant)
              n132 = Bundle By Name(cluster=T45 {"OCU Command"=enum."Add Global No-Sail", "Data"=variant}, "Data"=w340) -> (w341:T45)
              n133 = To Variant(anything=w341) -> (Variant=w339:variant)
              n134 = call "Write.vi"("error in (no error)"=w334, "element"=w339, "NetworkStreamWriter in"=w337) -> ("error out"=w338:errorcluster, "NetworkStreamWriter out"=w336:refnum<class "NetworkStreamWriter.lvclass">)  [unwired: 7 in]
            }
          }
        }
      }
      event "Reset Missions/Waypts": Value Change {
        n135 = event-data() -> ()  [unwired: 1 in, 1 out]
        n136 = case "Reset Missions" shown="True" "Reset Missions/Waypts" {
          tunnel: w357 -> [w361 w367]
          tunnel: w356 -> [w360 w366]
          tunnel: [w361 w365] -> w355
          tunnel: [w360 w364] -> w354
          frame False {
          }
          frame True {
            n137 = To Variant(anything=T45 {"OCU Command"=enum."Reset Missions/Waypts", "Data"=variant}) -> (Variant=w362:variant)
            n138 = call "Write.vi"("error in (no error)"=w366, "element"=w362, "NetworkStreamWriter in"=w367) -> ("error out"=w364:errorcluster, "NetworkStreamWriter out"=w365:refnum<class "NetworkStreamWriter.lvclass">)  [unwired: 7 in]
          }
        }
      }
      event Value Change {
        # "gray out the appropriate numeric controls"
        # "set input tool"
        # "Adjust OCU controls for the correct mission input style"
        n139 = event-data() -> ("NewVal"=w373:T4)  [unwired: 1 in]
        n140 = case shown="\"Station Keeping for\"" w373 {
          tunnel: [T47."Enabled" ("Disabled") w377 T47."Enabled" ("Disabled")] -> w372
          tunnel: [T47."Disabled and Grayed Out" ("Disabled") w377 T47."Enabled" ("Disabled")] -> w371
          frame "Go to Waypoint", Default {
          }
          frame "Pass Between Buoys", "Global No-Sail Zone" {
            w377 = T47."Disabled and Grayed Out" ("Disabled")
            # "\"Pass Between Buoys\"\nhas neither input"
          }
          frame "Station Keeping for" {
          }
        }
        n141 = case shown="\"Pass Between Buoys\", \"Global No-Sail Zone\"" w373 {
          tunnel: [w380 w381 w382] -> w374
          frame "Go to Waypoint", Default {
            w380 = u32 1 items=["Zoom Tool"=8, "Selection Tool"=0, "Pan Tool"=9, "Point Tool"=1, "Line Tool"=2, "Rectangle Tool"=3, "Rotated Rectangle Tool"=12, "Polyline Tool"=10, "Polygon Tool"=5, "Freehand Tool"=11, "Closed Freehand Tool"=6, "Ellipse Tool"=4, "Annulus Tool"=7] ("Current ROI Tool")
          }
          frame "Station Keeping for" {
            w381 = u32 2 items=["Zoom Tool"=8, "Selection Tool"=0, "Pan Tool"=9, "Point Tool"=1, "Line Tool"=2, "Rectangle Tool"=3, "Rotated Rectangle Tool"=12, "Polyline Tool"=10, "Polygon Tool"=5, "Freehand Tool"=11, "Closed Freehand Tool"=6, "Ellipse Tool"=4, "Annulus Tool"=7] ("Current ROI Tool")
          }
          frame "Pass Between Buoys", "Global No-Sail Zone" {
            w382 = u32 2 items=["Zoom Tool"=8, "Selection Tool"=0, "Pan Tool"=9, "Point Tool"=1, "Line Tool"=2, "Rectangle Tool"=3, "Rotated Rectangle Tool"=12, "Polyline Tool"=10, "Polygon Tool"=5, "Freehand Tool"=11, "Closed Freehand Tool"=6, "Ellipse Tool"=4, "Annulus Tool"=7] ("Current ROI Tool")
          }
        }
        n142 = property on="Tolerance" class="DigNum (strict)"("DisabledEnum"=w372) -> ()  [unwired: 2 in, 2 out]
        n143 = property on="Time(s)" class="DigNum (strict)"("DisabledEnum"=w371) -> ()  [unwired: 2 in, 2 out]
        n144 = property on="Mission Map"("Current ROI Tool"=w374) -> ()  [unwired: 2 in, 2 out]
      }
      event "Mission Map": Mouse Up {
        # "add a waypoint to the list"
        n145 = event-data() -> ()  [unwired: 1 in, 1 out]
        n146 = global read "OCUtoSim.vi" "Pause Simulator?"() -> (w383:bool)
        n147 = case shown="True" w383 {
          tunnel: w391 -> [w400 w523]
          tunnel: w390 -> [w399 w521]
          tunnel: [w398 w522] -> w389
          tunnel: [w397 w524] -> w388
          tunnel: w387 -> [w396 w524]
          tunnel: w386 -> [w395 _]
          tunnel: w385 -> [w394 _]
          tunnel: w384 -> [w393 _]
          frame False {
            n148 = case shown="\"Go to Waypoint\", Default" w395 {
              selector: w395 -> [_ _ w474 _ _]
              tunnel: w400 -> [w410 w436 w481 w499 w519]
              tunnel: [w408 w446 w478 w490 w510] -> w398
              tunnel: w399 -> [w409 w433 w463 w485 w517]
              tunnel: w394 -> [w403 _ w475 _ w500]
              tunnel: [w406 w444 w467 w493 w511] -> w397
              tunnel: w396 -> [w405 w443 w464 w494 w509]
              tunnel: w393 -> [_ _ _ _ w501]
              frame "Go to Waypoint", Default {
                n149 = property on="Mission Map"(error in=w410) -> (error out=w412:errorcluster, "Last Mouse Position"=w411)  [unwired: 1 in, 1 out]
                n150 = call "Helper - Image To UTM.vi"("Image Descriptor"=w409, "Pixel Coordinates"=w411) -> ("UTM Location"=w401:T15)  [unwired: 1 in, 1 out]
                n151 = invoke on="Mission Map" class="ImageControl" method="Clear ROI"(error in=w412) -> (error out=w407:errorcluster)  [unwired: 2 in, 2 out]
                n152 = disable-structure shown="Enabled" {
                  disable-tunnel: w403 -> [w419 w422]
                  disable-tunnel: [w415 w426] -> w402
                  disable-tunnel: w401 -> [w413 w421]
                  frame Enabled {
                    n153 = call "Initialize.vi"("Tolerance (m)"=w419, "Drive Location"=w413) -> ("Drive out"=w414:refnum<class "DriveTo.lvclass">)  [unwired: 8 in, 1 out]
                    n154 = Flatten To String(anything=w414) -> (data string=w416:string)  [unwired: 3 in, 2 out]
                    n155 = To Variant(anything=w416) -> (Variant=w417:variant)
                    n156 = Bundle By Name(cluster=T45 {"OCU Command"=enum."Add Mission", "Data"=variant}, "Data"=w417) -> (w415:T45)
                  }
                  frame Disabled {
                    n157 = call "init_waypoint.vi"("Coords"=w421, "Tolerance (m)"=w422) -> ("Waypoint Out"=w420:refnum<class "Waypoint.lvclass">)  [unwired: 9 in]
                    n158 = Flatten To String(anything=w420) -> (data string=w423:string)  [unwired: 3 in, 2 out]
                    n159 = To Variant(anything=w423) -> (Variant=w424:variant)
                    n160 = Bundle By Name(cluster=T45 {"OCU Command"=enum."Set waypoint number", "Data"=variant}, "Data"=w424) -> (w426:T45)
                  }
                }
                n161 = To Variant(anything=w402) -> (Variant=w404:variant)
                n162 = call "Write.vi"("error in (no error)"=w407, "element"=w404, "NetworkStreamWriter in"=w405) -> ("error out"=w408:errorcluster, "NetworkStreamWriter out"=w406:refnum<class "NetworkStreamWriter.lvclass">)  [unwired: 7 in]
              }
              frame "Global No-Sail Zone" {
                n163 = property on="Mission Map"(error in=w436) -> (error out=w435:errorcluster, "ROI"=w437)  [unwired: 1 in, 1 out]
                n164 = call "helper- line ROI to 2 UTM Pts.vi"("ROI"=w437, "Image Descriptor"=w433) -> ("Endpoint UTM 2"=w432:T15, "Endpoint UTM 1"=w434:T15)
                n165 = Unbundle By Name(w432) -> ("East"=w430:dbl, "North"=w431:dbl)
                n166 = Unbundle By Name(w434) -> ("UTM Zone"=w438:dbl, "Hemisphere"=w439:enum16{"North", "South"}, "East"=w428:dbl, "North"=w429:dbl)
                n167 = call "2 XYPointsToDistanceAndAngle.vi"("East 2"=w431, "North 2"=w430, "East 1"=w429, "North 1"=w428) -> ("Distance"=w427:dbl)  [unwired: 6 in, 1 out]
                n168 = invoke on="Mission Map" class="ImageControl" method="Clear ROI"(error in=w435) -> (error out=w445:errorcluster)  [unwired: 2 in, 2 out]
                n169 = disable-structure shown="Enabled" {
                  disable-tunnel: w427 -> [w452 w458]
                  disable-tunnel: [w454 w462] -> w441
                  disable-tunnel: T30 {"UTM Zone"=0.0, "Hemisphere"=enum."North", "East"=0.0, "North"=0.0, "Radius"=0.0} ("UTM Location") -> [w453 _]
                  disable-tunnel: w429 -> [w451 _]
                  disable-tunnel: w428 -> [w450 _]
                  disable-tunnel: w439 -> [w449 _]
                  disable-tunnel: w438 -> [w448 _]
                  frame Enabled {
                    n170 = Bundle By Name(cluster=w453, "UTM Zone"=w448, "Hemisphere"=w449, "East"=w450, "North"=w451, "Radius"=w452) -> (w447:T30)
                    n171 = To Variant(anything=w447) -> (Variant=w455:variant)
                    n172 = Bundle By Name(cluster=T45 {"OCU Command"=enum."Add Global No-Sail", "Data"=variant}, "Data"=w455) -> (w454:T45)
                  }
                  frame Disabled {
                    n173 = call "init_waypoint.vi"("Tolerance (m)"=w458) -> ("Waypoint Out"=w457:refnum<class "Waypoint.lvclass">)  [unwired: 10 in]
                    n174 = Flatten To String(anything=w457) -> (data string=w459:string)  [unwired: 3 in, 2 out]
                    n175 = To Variant(anything=w459) -> (Variant=w460:variant)
                    n176 = Bundle By Name(cluster=T45 {"OCU Command"=enum."Set waypoint number", "Data"=variant}, "Data"=w460) -> (w462:T45)
                  }
                }
                n177 = To Variant(anything=w441) -> (Variant=w442:variant)
                n178 = call "Write.vi"("error in (no error)"=w445, "element"=w442, "NetworkStreamWriter in"=w443) -> ("error out"=w446:errorcluster, "NetworkStreamWriter out"=w444:refnum<class "NetworkStreamWriter.lvclass">)  [unwired: 7 in]
              }
              frame "Round Buoy Starboard", "Round Buoy Port" {
                n179 = property on="Mission Map"(error in=w481) -> (error out=w483:errorcluster, "Last Mouse Position"=w482)  [unwired: 1 in, 1 out]
                n180 = Equal?(x=w474, y=Mission_Type_Radio_Buttons."Round Buoy Port" ("Mission Type 2")) -> (x = y?=w469:bool)
                n181 = call "Helper - Image To UTM.vi"("Image Descriptor"=w463, "Pixel Coordinates"=w482) -> ("UTM Location"=w476:T15)  [unwired: 1 in, 1 out]
                n182 = invoke on="Mission Map" class="ImageControl" method="Clear ROI"(error in=w483) -> (error out=w478:errorcluster)  [unwired: 2 in, 2 out]
                n183 = Select(t=enum16{"Starboard", "Port"}."Port" ("Round side?"), s=w469, f=enum16{"Starboard", "Port"}."Starboard" ("Round side?")) -> (s? t:f=w470:enum16{"Starboard", "Port"})
                n184 = call "Initialize.vi"("Tolerance (m)"=w475, "Round side?"=w470, "Buoy to Round"=w476) -> ("RoundBuoys out"=w468:refnum<class "RoundBuoy.lvclass">)  [unwired: 7 in, 1 out]
                n185 = Flatten To String(anything=w468) -> (data string=w477:string)  [unwired: 3 in, 2 out]
                n186 = To Variant(anything=w477) -> (Variant=w479:variant)
                n187 = Bundle By Name(cluster=T45 {"OCU Command"=enum."Add Mission", "Data"=variant}, "Data"=w479) -> (w465:T45)
                n188 = To Variant(anything=w465) -> (Variant=w466:variant)
                n189 = call "Write.vi"("element"=w466, "NetworkStreamWriter in"=w464) -> ("NetworkStreamWriter out"=w467:refnum<class "NetworkStreamWriter.lvclass">)  [unwired: 8 in, 1 out]
              }
              frame "Pass Between Buoys" {
                # "build Pass Between Buoys mission"
                n190 = property on="Mission Map"(error in=w499) -> (error out=w491:errorcluster, "ROI"=w484)  [unwired: 1 in, 1 out]
                n191 = invoke on="Mission Map" class="ImageControl" method="Clear ROI"(error in=w491) -> (error out=w492:errorcluster)  [unwired: 2 in, 2 out]
                n192 = call "helper- line ROI to 2 UTM Pts.vi"("ROI"=w484, "Image Descriptor"=w485) -> ("Endpoint UTM 2"=w487:T15, "Endpoint UTM 1"=w486:T15)
                n193 = call "Initialize.vi"("Buoy Pass 2"=w487, "Buoy Pass 1"=w486) -> ("PassBuoys out"=w488:refnum<class "PassBuoys.lvclass">)  [unwired: 8 in, 1 out]
                n194 = Flatten To String(anything=w488) -> (data string=w496:string)  [unwired: 3 in, 2 out]
                n195 = To Variant(anything=w496) -> (Variant=w497:variant)
                n196 = Bundle By Name(cluster=T45 {"OCU Command"=enum."Add Mission", "Data"=variant}, "Data"=w497) -> (w495:T45)
                n197 = To Variant(anything=w495) -> (Variant=w489:variant)
                n198 = call "Write.vi"("error in (no error)"=w492, "element"=w489, "NetworkStreamWriter in"=w494) -> ("error out"=w490:errorcluster, "NetworkStreamWriter out"=w493:refnum<class "NetworkStreamWriter.lvclass">)  [unwired: 7 in]
              }
              frame "Station Keeping for" {
                # "user inputs two points as a line and we convert it to a square"
                n199 = property on="Mission Map"(error in=w519) -> (error out=w507:errorcluster, "ROI"=w518)  [unwired: 1 in, 1 out]
                n200 = call "helper- line ROI to 2 UTM Pts.vi"("ROI"=w518, "Image Descriptor"=w517) -> ("Endpoint UTM 2"=w502:T15, "Endpoint UTM 1"=w503:T15)
                n201 = call "helper - UTM line to Square.vi"("Endpoint 2, UTM"=w502, "Endpoint 1, UTM"=w503) -> ("Endpoint 4, UTM"=w505:T15, "Endpoint 3, UTM"=w504:T15)
                n202 = invoke on="Mission Map" class="ImageControl" method="Clear ROI"(error in=w507) -> (error out=w508:errorcluster)  [unwired: 2 in, 2 out]
                n203 = call "Initialize.vi"("Tolerance (m)"=w500, "Duration (s)"=w501, "Buoy SE"=w502, "Buoy SW"=w503, "Buoy NE"=w505, "Buoy NW"=w504) -> ("StationKeeping out"=w506:refnum<class "StationKeeping.lvclass">)  [unwired: 4 in, 1 out]
                n204 = Flatten To String(anything=w506) -> (data string=w514:string)  [unwired: 3 in, 2 out]
                n205 = To Variant(anything=w514) -> (Variant=w515:variant)
                n206 = Bundle By Name(cluster=T45 {"OCU Command"=enum."Add Mission", "Data"=variant}, "Data"=w515) -> (w513:T45)
                n207 = To Variant(anything=w513) -> (Variant=w512:variant)
                n208 = call "Write.vi"("error in (no error)"=w508, "element"=w512, "NetworkStreamWriter in"=w509) -> ("error out"=w510:errorcluster, "NetworkStreamWriter out"=w511:refnum<class "NetworkStreamWriter.lvclass">)  [unwired: 7 in]
              }
            }
          }
          frame True {
            # "While we're paused, if you click on the map, that sets the new location and flushes velocity/rate of turn"
            n209 = global read "OCUtoSim.vi" "Move boat?"() -> (w520:bool)
            n210 = case shown="True" w520 {
              tunnel: w523 -> [w525 w532]
              tunnel: [w525 w531] -> w522
              tunnel: w521 -> [_ w528]
              frame False {
              }
              frame True {
                n211 = property on="Mission Map"(error in=w532) -> (error out=w533:errorcluster, "Last Mouse Position"=w530)  [unwired: 1 in, 1 out]
                n212 = invoke on="Mission Map" class="ImageControl" method="Clear ROI"(error in=w533) -> (error out=w531:errorcluster)  [unwired: 2 in, 2 out]
                n213 = call "Helper - Image To UTM.vi"("Image Descriptor"=w528, "Pixel Coordinates"=w530) -> ("UTM Location"=w529:T15)  [unwired: 1 in, 1 out]
                n214 = global write "2 Global.vi" "Robot\nRate of Turn"(T17 0.0 ("Robot\nRate of Turn")) -> ()
                n215 = global write "2 Global.vi" "Robot UTM Location"(w529) -> ()
                n216 = global write "2 Global.vi" "Robot Velocity"(T16 {"East"=0.0, "North"=0.0} ("Robot Velocity")) -> ()
              }
            }
          }
        }
      }
      event "Pause Simulator?": Value Change {
        # "Why are there so many controls......."
        # "I'm leaving the tuning constants\nas is because they'll change anyway."
        # "Disable controls when paused because it doesn't make sense to change them while paused!"
        n217 = event-data() -> ("NewVal"=w535:bool)  [unwired: 1 in, 1 out]
        n218 = case shown="True" w534 {
          tunnel: w535 -> [_ w539]
          frame False {
          }
          frame True {
            n219 = global write "OCUtoSim.vi" "Pause Simulator?"(w539) -> ()
            n220 = Select(t=T47."Disabled and Grayed Out" ("Disabled"), s=w539, f=T47."Enabled" ("Disabled")) -> (s? t:f=w540:T47)
            n221 = property on="OVERRIDE RUDDER?" class="Bool (strict)"("DisabledEnum"=w540) -> ()  [unwired: 2 in, 2 out]
            n222 = property on="OVERRIDE SAIL?" class="Bool (strict)"("DisabledEnum"=w540) -> ()  [unwired: 2 in, 2 out]
            n223 = property on="Load MDF" class="Bool"("DisabledEnum"=w540) -> ()  [unwired: 2 in, 2 out]
            n224 = property on="Location of THINK" class="CmbBox (strict)"("DisabledEnum"=w540) -> ()  [unwired: 2 in, 2 out]
            n225 = property on="Map Name" class="CmbBox (strict)"("DisabledEnum"=w540) -> ()  [unwired: 2 in, 2 out]
            n226 = property on="Mission Def Filepath" class="Path"("DisabledEnum"=w540) -> ()  [unwired: 2 in, 2 out]
            n227 = property on="Setpoints to boat" class="Clust (strict)"("DisabledEnum"=w540) -> ()  [unwired: 2 in, 2 out]
            n228 = property on="Mission Entry Type" class="RadioBtnsControl (strict)"("DisabledEnum"=w540) -> ()  [unwired: 2 in, 2 out]
          }
        }
      }
      event "Set Wind Speed": Value Change {
        # "Control the wind speed for the simulator from the OCU.\nTechnically pause simulator should never be true when it's not the simulator.\nBut do you really want to risk it?"
        n229 = event-data() -> ("NewVal"=w550:dbl)  [unwired: 1 in, 1 out]
        n230 = global read "OCUtoSim.vi" "Pause Simulator?"() -> (w547:bool)
        n231 = Not(x=w547) -> (.not. x?=w546:bool)
        n232 = And(x=w548, y=w546) -> (x .and. y?=w549:bool)
        n233 = case shown="True" w549 {
          tunnel: w550 -> [_ w551]
          frame False {
          }
          frame True {
            n234 = global write "2 Global.vi" "Absolute Wind\nSpeed"(w551) -> ()
          }
        }
      }
      event "Set Wind Direction": Value Change {
        # "If we're on the simulator AND it isn't paused, let us change\nthe wind direction."
        n235 = event-data() -> ("NewVal"=w555:dbl)  [unwired: 1 in, 1 out]
        n236 = global read "OCUtoSim.vi" "Pause Simulator?"() -> (w557:bool)
        n237 = Not(x=w557) -> (.not. x?=w559:bool)
        n238 = And(x=w558, y=w559) -> (x .and. y?=w556:bool)
        n239 = case shown="True" w556 {
          tunnel: w555 -> [_ w560]
          frame False {
          }
          frame True {
            n240 = global write "2 Global.vi" "Absolute Wind\nDirection (º)"(w560) -> ()
          }
        }
      }
      event "Set Water Current Speed", "Set Water Current Direction": Value Change {
        # "set the water current based on the controls. Angles correspond to how they look on the dial."
        n241 = event-data() -> ()  [unwired: 1 in, 1 out]
        n242 = case "Only allow water current to be set in simulation." shown="True" w561 {
          frame False {
          }
          frame True {
            n243 = global read "2 Global.vi" "Absolute Water Current Vector"() -> (w572:T19)
            n244 = expression code="(x/180.0)*pi" "degrees to radians"("Set Water Current Direction") -> (w570:dbl)
            n245 = Cosine(x=w570) -> (cos(x)=w568:dbl)
            n246 = Sine(x=w570) -> (sin(x)=w569:dbl)
            n247 = Multiply(x="Set Water Current Speed", y=w568) -> (x*y=w565:dbl)
            n248 = Multiply(x=w569, y="Set Water Current Speed") -> (x*y=w566:dbl)
            n249 = Bundle By Name(cluster=w572, "North"=w566, "East"=w565) -> (w573:T19)
            n250 = global write "2 Global.vi" "Absolute Water Current Vector"(w573) -> ()
          }
        }
      }
      event "Move boat?": Value Change {
        # "If we're on the simulator, and we're pausing the simulator, and we want to move the boat, let us move the boat."
        n251 = event-data() -> ("NewVal"=w580:bool)  [unwired: 1 in, 1 out]
        n252 = global read "OCUtoSim.vi" "Pause Simulator?"() -> (w577:bool)
        n253 = Compound Arithmetic op=AND(w580, w577, w578) -> (w579:bool)
        n254 = global write "OCUtoSim.vi" "Move boat?"(w579) -> ()
      }
      event "Set Boat Heading": Value Change {
        n255 = event-data() -> ("NewVal"=w584:dbl)  [unwired: 1 in, 1 out]
        n256 = global read "OCUtoSim.vi" "Move boat?"() -> (w587:bool)
        n257 = global read "OCUtoSim.vi" "Pause Simulator?"() -> (w586:bool)
        n258 = Compound Arithmetic op=AND(w588, w587, w586) -> (w585:bool)
        n259 = case shown="True" w585 {
          tunnel: w584 -> [_ w589]
          frame False {
          }
          frame True {
            n260 = global write "2 Global.vi" "Robot\nHeading"(w589) -> ()
          }
        }
      }
    }
    n261 = local read "Setpoints to boat"() -> (w50:T23)
    n262 = local read "OVERRIDE RUDDER?"() -> (w55:bool)
    n263 = local read "OVERRIDE SAIL?"() -> (w51:bool)
    n264 = Unbundle By Name(w57) -> ("Sail Position"=w52:T24, "Rudder Angle"=w53:T25)
    n265 = Unbundle By Name(w50) -> ("Sail Position"=w49:T24, "Rudder Angle"=w48:T25)
    n266 = call "eStopShared.vi"("Command"=eStopCommand."Set E-Stop", "E-Stop"="Stop") -> ("E-Stop Out"=w62:bool)  [unwired: 8 in, 1 out]
    n267 = Not Equal?(x=w38, y=T11 "192.168.1.6") -> ()  [unwired: 1 out]
    n268 = Select(t=w52, s=w51, f=w49) -> (s? t:f=w40:T24)
    n269 = Select(t=w53, s=w55, f=w48) -> (s? t:f=→"Rudder Position":T25)
    n270 = case "Chaos and sim both have 180\ndegrees of motion in sail" shown="False" FALSE {
      tunnel: w40 -> [w68 w69]
      tunnel: [w65 w69] -> w39
      frame False {
        n271 = In Range and Coerce(upper limit=T24 1.0, x=w68, lower limit=T24 0.0) -> (coerced(x)=w65:T24)  [unwired: 1 out]
      }
      frame True {
      }
    }
    "Sail Position 2" <- w39
  }
  n272 = while "Read from network stream to update" {
    shift-right: [w647] -> w29
    shift-left: w32 -> [w642]
    shift-right: [w640] -> w28
    shift-left: w6 -> [w641]
    tunnel: w27 -> [w644]
    tunnel: w14 -> [w643]
    stop <- w645 stop-if-true
    n273 = call "IsConnected.vi"("error in (no error)"=w641, "NetworkStreamReader in"=w642) -> ("error out"=w636:errorcluster, "Connected?"=→"Connected?":bool, "NetworkStreamReader out"=w637:refnum<class "NetworkStreamReader.lvclass">)  [unwired: 7 in]
    n274 = call "Read.vi"("Read Type"=readType."Most current", "error in (no error)"=w636, "NetworkStreamReader in"=w637) -> ("error out"=w633:errorcluster, "element"=w632:variant, "NetworkStreamReader out"=w647:refnum<class "NetworkStreamReader.lvclass">)  [unwired: 4 in, 2 out]
    n275 = Variant To Data(error in=w633, type=T36 {"Sensor Status"={"Sensor Connected"=FALSE, "Sensor Initialized"=FALSE, "Sensor OK"=FALSE, "Latest Error String"="", "GPS Lock"=FALSE}, "Battery Voltage"=0.0, "Rudder Actuator Status"={"Actuator Connected"=FALSE}, "Sail Actuator Status"={"Actuator Connected"=FALSE}, "Which Boat Am I?"=enum."Axiom; Blackbody Radiation", "Robot Velocity"={"East"=0.0, "North"=0.0}, "Robot UTM Location"={"UTM Zone"=0.0, "Hemisphere"=enum."North", "East"=0.0, "North"=0.0}, "Robot\nHeading "=0.0, "Robot\nRate of Turn"=0.0, "Robot Pitch/Roll"={"Pitch"=0.0, "Roll"=0.0}, "Apparent Wind"={"Toward Fore"=0.0, "Toward Starboard"=0.0}, "Apparent Wind\nSpeed"=0.0, "Apparent Wind\nDirection (º)"=0.0, "Absolute Wind"={"East"=0.0, "North"=0.0}, "Absolute Wind\nDirection (º)"=0.0, "Absolute Wind\nSpeed"=0.0, "Absolute Water Current Vector"={"Direction"=0.0, "Magnitude"=0.0}, "Rudder Angle"=0.0, "Sail Position"=0.0, "Manual Override Cluster"={"Override Active Rudder"=FALSE, "Setpoints"={"Sail Position"=0.0, "Rudder Angle"=0.0}, "Override Active Sail"=FALSE}, "Setpoints to boat"={"Sail Position"=0.0, "Rudder Angle"=0.0}, "Current Waypoint"=0, "Think freq."=0.0, "Sense freq."=0.0, "Act freq."=0.0, "E-stop freq."=0.0, "Network \nfreq."=0.0, "Network \nLoop Iterations"=0, "E-Stop"=FALSE, "Serialized Waypoint Array"="", "Serialized Mission Queue Elements"="", "Goodness Functions"={0.0, 0.0, []}, "Global No Sail Circles"=[], "Optimal Heading"=0.0, "Crossing Wind"=FALSE, "Estimated Error"=0.0, "Don't Tip?"=FALSE, "Tacking Attempt"={"attempting tack"=FALSE, "tacking attempt\ntime remaining"=0.0}} ("RIO->OCU update data"), Variant=w632) -> (data=w630:T36, error out=w635:errorcluster)
    n276 = Unbundle By Name(w630) -> ("Estimated Error"=→"Estimated Error":dbl, "Sensor Status"=→"Wind Sensor Status":T12, "Battery Voltage"=→"Battery Voltage":dbl, "Which Boat Am I?"=→"You are sailing":T5, "Robot Velocity"=w598:T16, "Robot UTM Location"=w610:T15, "Robot\nHeading"=w606:T8, "Robot\nRate of Turn"=→"Robot\nRate of Turn":T17, "Robot Pitch/Roll"=→"Robot Pitch/Roll":T18, "Absolute Wind\nDirection (º)"=→"Absolute\nWind\nDirection":T38, "Apparent Wind"=→"Apparent Wind":T22, "Apparent Wind\nSpeed"=→"Apparent Wind Speed":T21, "Apparent Wind\nDirection (º)"=→"Apparent Wind Direction" →"Apparent Wind Direction\nPoint of Sail":T20, "Absolute Wind"=→"Absolute Wind":T19, "Rudder Angle"=→"Rudder Angle":T25, "Sail Position"=w621:T24, "Manual Override Cluster"=→"Manual Override":T27, "Setpoints to boat"=→"Setpoints to boat":T23, "Serialized Mission Queue Elements"=w617:string, "Global No Sail Circles"=w614:T30[], "Optimal Heading"=w609:dbl, "Goodness Functions"=w613:T41, "Current Waypoint"=w600:T26, "Serialized Waypoint Array"=w620:string, "Crossing Wind"=→"Crossing Wind":bool, "Don't Tip?"=→"Don't Tip?":bool)  [unwired: 6 out]
    "Robot UTM Location" <- w610
    "Robot Heading" <- w606
    "Robot Velocity" <- w598
    "Sail Position" <- w621
    "Current Waypoint" <- w600
    "Global No Sail Circles" <- w614
    "Heading" <- w606
    n277 = global read "2 Global.vi" "Absolute Wind\nDirection (º)"() -> (→"Local Wind":T38)
    n278 = Bundle("Image Ref Out"=w644, "Image Descriptor"=w643) -> (w608:T50)  [unwired: 1 in]
    n279 = call "Deserialize Waypoint Array.vi"("Serialized Waypoint Array"=w620) -> ("Waypoints Object Array"=w618:T29, "Waypoints Array"=→"Waypoints Array":T28[])  [unwired: 9 in]
    "Waypoints Object Array" <- w618
    n280 = call "deserializeMissionArray.vi"("Serialized Mission Array"=w617) -> ("Mission Object Array"=w601:refnum<class "GenericMission.lvclass">[])  [unwired: 9 in, 1 out]
    "Mission Object Array" <- w601
    n281 = call "Velocity Converter- dx-dy to magnitude-heading.vi"("Vector In"=w598) -> ("Magnitude Out"=→"Robot Speed (m/s)":dbl)  [unwired: 9 in, 1 out]
    n282 = call "0-Do Overlays.vi"("Image Reference\nand Descriptor"=w608, "Missions"=w601, "No Sail Circles"=w614, "Waypoints"=w618, "Current Waypoint #"=w600, "Heading"=w606, "Sail Position"=w621, "Robot UTM Location"=w610, "Optimal Heading"=w609, "Font Size"="Overlay Font Size") -> ("Image out"=→"Mission Map":T7)  [unwired: 5 in]
    n283 = Array Size(array=w618) -> (size(s)=→"# of Waypts":i32)
    n284 = call "Helper - goodness polar plot.vi"("Plot Colors"="Plot Colors", "Goodness Fns In"=w613) -> ("Goodness Functions Polar Plot"=→"Goodness Functions":picture)  [unwired: 9 in]
    n285 = Index Array(array=w601, index=0) -> (element=w602:refnum<class "GenericMission.lvclass">)
    n286 = call-dynamic "getStatus.vi"("GenericMission in"=w602) -> ("Status"=→"Mission Status":string)  [unwired: 8 in, 2 out]
    n287 = Wait (ms)(milliseconds to wait=u32 50 ("millisecond multiple")) -> ()  [unwired: 1 out]
    n288 = call "eStopShared.vi"("Command"=eStopCommand."Get E-Stop", "Error In"=w635) -> ("Error Out"=w640:errorcluster, "E-Stop Out"=w645:bool)  [unwired: 8 in]
  }
  n289 = while {
    stop <- w657 stop-if-true
    n290 = global read "2 Global.vi" "Sensor Status"() -> (w655:T12)
    "Sensor Status" <- w655
    n291 = Unbundle By Name(w655) -> ("Sensor OK"=w651:T13, "Sensor Initialized"=w650:T13, "GPS Lock"=w648:T13)
    n292 = And(x=w651, y=w650) -> (x .and. y?=w649:T13)
    n293 = case shown="True" "Enable \nLocal GPS" {
      tunnel: w649 -> [_ w660]
      frame False {
        n294 = Wait Until Next ms Multiple(millisecond multiple=u32 100) -> ()  [unwired: 1 out]
      }
      frame True {
        n295 = case shown="False" w660 {
          tunnel: [w667 w669] -> w664
          tunnel: "GPS COM port" -> [w668 w669]
          tunnel: [w666 _] -> w662
          frame False {
            n296 = call "1A Helper - Init Sensor.vi"("VISA Refnum in"=w668) -> ("error out"=w666:errorcluster, "VISA Refnum out"=w667:refnum<visa-resource-name>)  [unwired: 8 in, 1 out]
          }
          frame True {
          }
        }
        n297 = call "1A Read Sensor Data.vi"("error (in)"=w662, "VISA resource name (in)"=w664) -> ("error (out)"=w661:errorcluster)  [unwired: 8 in, 1 out]
        n298 = case shown="Error" w661 {
          frame No Error {
          }
          frame Error {
            n299 = local write "Enable \nLocal GPS"(FALSE ("Enable \nLocal GPS")) -> ()
          }
        }
      }
    }
    n300 = call "eStopShared.vi"("Command"=eStopCommand."Get E-Stop") -> ("E-Stop Out"=w657:bool)  [unwired: 9 in, 1 out]
    n301 = Select(t=T47."Enabled" ("Disabled"), s=w648, f=T47."Disabled and Grayed Out" ("Disabled")) -> (s? t:f=w652:T47)
    n302 = property on="Local to Point 0" class="Bool"("DisabledEnum"=w652) -> ()  [unwired: 2 in, 2 out]
    n303 = property on="Local to Point 1" class="Bool"("DisabledEnum"=w652) -> ()  [unwired: 2 in, 2 out]
    n304 = property on="Local to Point 2" class="Bool"("DisabledEnum"=w652) -> ()  [unwired: 2 in, 2 out]
    n305 = property on="Local to Point 3" class="Bool"("DisabledEnum"=w652) -> ()  [unwired: 2 in, 2 out]
    n306 = property on="Local to Point 4" class="Bool"("DisabledEnum"=w652) -> ()  [unwired: 2 in, 2 out]
  }
  n307 = call "Close.vi"("error in (no error)"=w28, "NetworkStreamReader in"=w29) -> ()  [unwired: 9 in, 1 out]
  n308 = call "Close.vi"("error in (no error)"=w23, "NetworkStreamWriter in"=w24) -> ()  [unwired: 9 in, 1 out]
